vi "MAIN_5.3.vi"() -> ()   [LabVIEW 2012]
doc: "Use this template to build a producer/consumer design pattern with events to produce queue items. Use this design pattern instead of the User Interface Event Handler pattern for user interfaces when you want to execute code asynchronously in response to an event without slowing the user interface responsiveness."
uses:
  State_machine_enum.ctl
  display2.ctl
  User_buttons_enum.ctl
  <vilib>/DAQmx/read.llb/DAQmx Read (Analog 2D DBL NChan NSamp).vi
  Global 1_diag.vi
  <vilib>/Waveform/WDTFileIO.llb/Export Waveforms To Spreadsheet File (1D).vi
  <vilib>/Utility/file.llb/Write To Spreadsheet File (DBL).vi
  <vilib>/DAQmx/create/channels.llb/DAQmx Create Channel (AI-Voltage-Basic).vi
  <vilib>/DAQmx/configure/timing.llb/DAQmx Timing (Sample Clock).vi
  <vilib>/DAQmx/miscellaneous.llb/DAQmx Fill In Error Info.vi
  <vilib>/Analysis/baseanly.llb/Mean (DBL).vi
  <vilib>/express/express arith-compare/Formula/XNode/ExpressFormulaBlockNode.xnode
  <vilib>/Analysis/NI_AALBase.lvlib
  <resource>/objmgr/daqmx.rc
panel:
  out "LD(cont/disc)":T1
  out "LD error array disc":dbl[](array[numeric])
  out "LD array disc":dbl[](array[numeric])
  in  "Timetrace save":bool
  out "result":bool=TRUE
  out "dt":dbl=0.001
  in  "Lock In":bool
  out "dLD_RMS":dbl=nan
  out "Waveform Graph":waveform(dbl)[](graph)=[{"t0"=timestamp(0 s since 1904-01-01), "dt"=0.001, "Y"=[]}, {"t0"=timestamp(0 s since 1904-01-01), "dt"=0.001, "Y"=[]}]
  out "error out":errorcluster
  out "Unbalanced?":bool
  in  "Second Harmonic":bool
  out "path":path
  out "Signal Balance":bool
  out "DC Voltage (V) 2":dbl(knob)=nan scale=0.0..10.0
  out "2f Frequency (Hz)":dbl(knob)=-inf scale=0.0..150.0
  in  "Voltage Divider (10)":bool
  out "Actual Task":string="Plotting"
  out "Motor Voltage (V)":dbl=1.0
  in  "Initial Voltage (V)":dbl=0.35 min=0.0 max=9.0
  in  "Final Voltage (V)":dbl=1.4 min=0.0 max=2.0
  in  "Voltage Step (V)":dbl=0.1 min=0.0 max=1000.0
  in  "Motor Stabilization Time (s)":dbl(knob)=10.0 step=0.001 scale=0.0..30.0
  out "Initial Voltage (V) 2":dbl=1.4 min=0.0 max=9.0
  in  "Final Voltage (V) 2":dbl=4.0 min=0.0 max=2.0
  in  "Voltage Step (V) 2":dbl=0.2 min=0.0 max=1000.0
  in  "Comment (sample no)":string
  in  "Stop Measurement":bool
  in  "Start Measurement Button":bool
  out "Measurement File":path
  in  "New File":bool
  out "Reset?":bool=TRUE
  out "Actual State":T2=enum."Measure"
  in  "Tab Control":T3(tab)=enum."Options"
  in  "Convert mld":bool
  in  "Convert parasiteno":bool
  in  "Convert parasitemia":bool
  in  "Convert cc":bool
  out "MLD (mV/V)":dbl=0.24515589898324114 format="%#_3g"
  out "SA 1f (mv/V)":dbl
  out "Lock_in (mV/V)":dbl
  out "dLock_in (mV/V)":dbl
  out "dMLD (mV/V)":dbl=0.05171335185673877 format="%#_3g"
  out "Phase (deg)":dbl=-68.05035522636679 format="%0.2f"
  out "Phase  dev (deg)":dbl=5.540360076813409 format="%0.2f"
  out "SA 2f (mv/V)":dbl
  out "MLD Amplitude (mV/V)":cluster{dbl[], dbl[]}[](graph)
  in  "dT/T (%)":dbl
  in  "Dilution":dbl=20.0
  in  "Undiluted cc.\n (ng/ml)":dbl
  in  "Undiluted \nParasitemia (%)":dbl format="%#_6f"
  in  "Parasites/ul\nof Blood":dbl
  in  "Convert dT":bool
  in  "MLD (mV/V)":dbl
  out "MLD Phase":cluster{dbl[], dbl[]}(graph)
  out "Down":bool
  out "Up":bool
  out "2f Frequency (Hz)":T4=-inf format="%0.3f"
  out "1f SA (mV/V)":T4 format="%0.3f"
  out "MLD Sim. LIA (mV/V)":T4=nan format="%0.3f"
  out "MLD SA (mV/V)":T4 format="%0.3f"
  in  "Start Scope":bool
  in  "Constant Motor Voltage":dbl=1.0
  in  "Refresh in (s)":i8=1
  in  "stop":bool
  in  "AC?":bool
  out "levelB":dbl format="%#_2g"
  out "levelA":dbl format="%#_3g"
  in  "V/div B":dbl(knob)=0.2 scale=10.0..0.01 scale format="%#_3g"
  in  "level B":dbl(slide) scale=-1.0..1.0 scale format="%#_3g"
  in  "level A":dbl(slide) scale=-1.0..1.0 scale format="%#_3g"
  in  "V/div A":dbl(knob)=0.2 scale=10.0..0.01 scale format="%#.3f"
  out "Oscilloscope":waveform(dbl)[](graph)=[{"t0"=timestamp(0 s since 1904-01-01), "dt"=0.001, "Y"=[]}, {"t0"=timestamp(0 s since 1904-01-01), "dt"=0.001, "Y"=[]}]
  in  "Sensitivity":T5(ring)
  in  "samples per channel":i32=1000
  in  "rate":dbl=1000.0 format="%0.2f"
  out "Spectrum (mVRMS/Vdc)":cluster{"f0":dbl, "df":dbl, "magnitude":dbl[]}(graph)={"f0"=0.0, "df"=inf, "magnitude"=[]}
  out "MLD LIA (mV/V)":dbl=0.0123978
  out "Lockin_freq":dbl=9.4676
  out "DC Voltage (V)":T4=nan format="%0.3f"
  out "Time Domain Signal":cluster{"xi used":dbl[], "yi":dbl[]}[](graph)
  out "Signal Spectrum (mVrms/Vdc)":cluster{"f0":dbl, "df":dbl, "magnitude":dbl[]}[](graph)
  out "1f 2f Spectral Peaks":T6
  out "Lock-in R (Vrms)":cluster{dbl[], "Result":dbl[]}(graph)
  out "Lock-in Theta":cluster{dbl[], "Result":dbl[]}(graph)
  in  "Pike Removal (StDev)":dbl=3.0
  in  "Lock-in Time (s)":dbl=10.0
  in  "dt (s)":dbl=0.0002
  in  "Resolution (s)":dbl=0.0001
  in  "Averaging time (s)":dbl=1.0 format="%0.2p"
  in  "Cutoff Frequency (Hz)":dbl=500.0
  in  "Rate":dbl=5000.0 caption="Sample Rate (Hz)" format="%0.2f"
  in  "Samples per Channel":i32=100000
  out "Minimum Value":dbl=-1.0 caption="LD min Value (V)" format="%0.2f"
  out "Maximum Value":dbl=1.0 caption="LD max Value (V)" format="%0.2f"
  in  "DC # samples":i32=100
  in  "DC Sampling Rate (Hz)":dbl=100.0
  in  "Dc min":dbl format="%0.2f"
  in  "Dc max":dbl=10.0 format="%0.2f"
  in  "Reference Signal":tag="Dev3/ai1"
  in  "LD Signal":tag="Dev3/ai0" caption="LD Channel"
  in  "DC Voltage DAQ":tag="Dev3/ai2"
  in  "Motor Channel":tag="Dev3/ao1"
  in  "Lock-in-Amplifier VISA":refnum<visa-resource-name>="GPIB0::3::INSTR"
  out "Dc standard deviation":dbl=-0.0 format="%0.2f"
  out "Dc mean":dbl=nan format="%0.2f"
  out "dPhase array":dbl[](array[numeric])
  out "Phase array":dbl[](array[numeric])
  out "LD array":dbl[](array[numeric])
  out "Frequency array":dbl[](array[numeric])
  out "LD error array":dbl[](array[numeric])
  out "First?":bool
  out "Stopped":bool
  out "Last Step?":bool
  in  "EXIT":bool
  # "Measurement Settings"
  # "Motor Setup"
  # "OFF"
  # "ON"
  # "Actual Datapoint Values"
  # "Convert quantities"
  # "Physical channels"
  # "Signal Processing Settings"
  # "DC Acquisition Settings"
  # "LD Acquisition Settings"
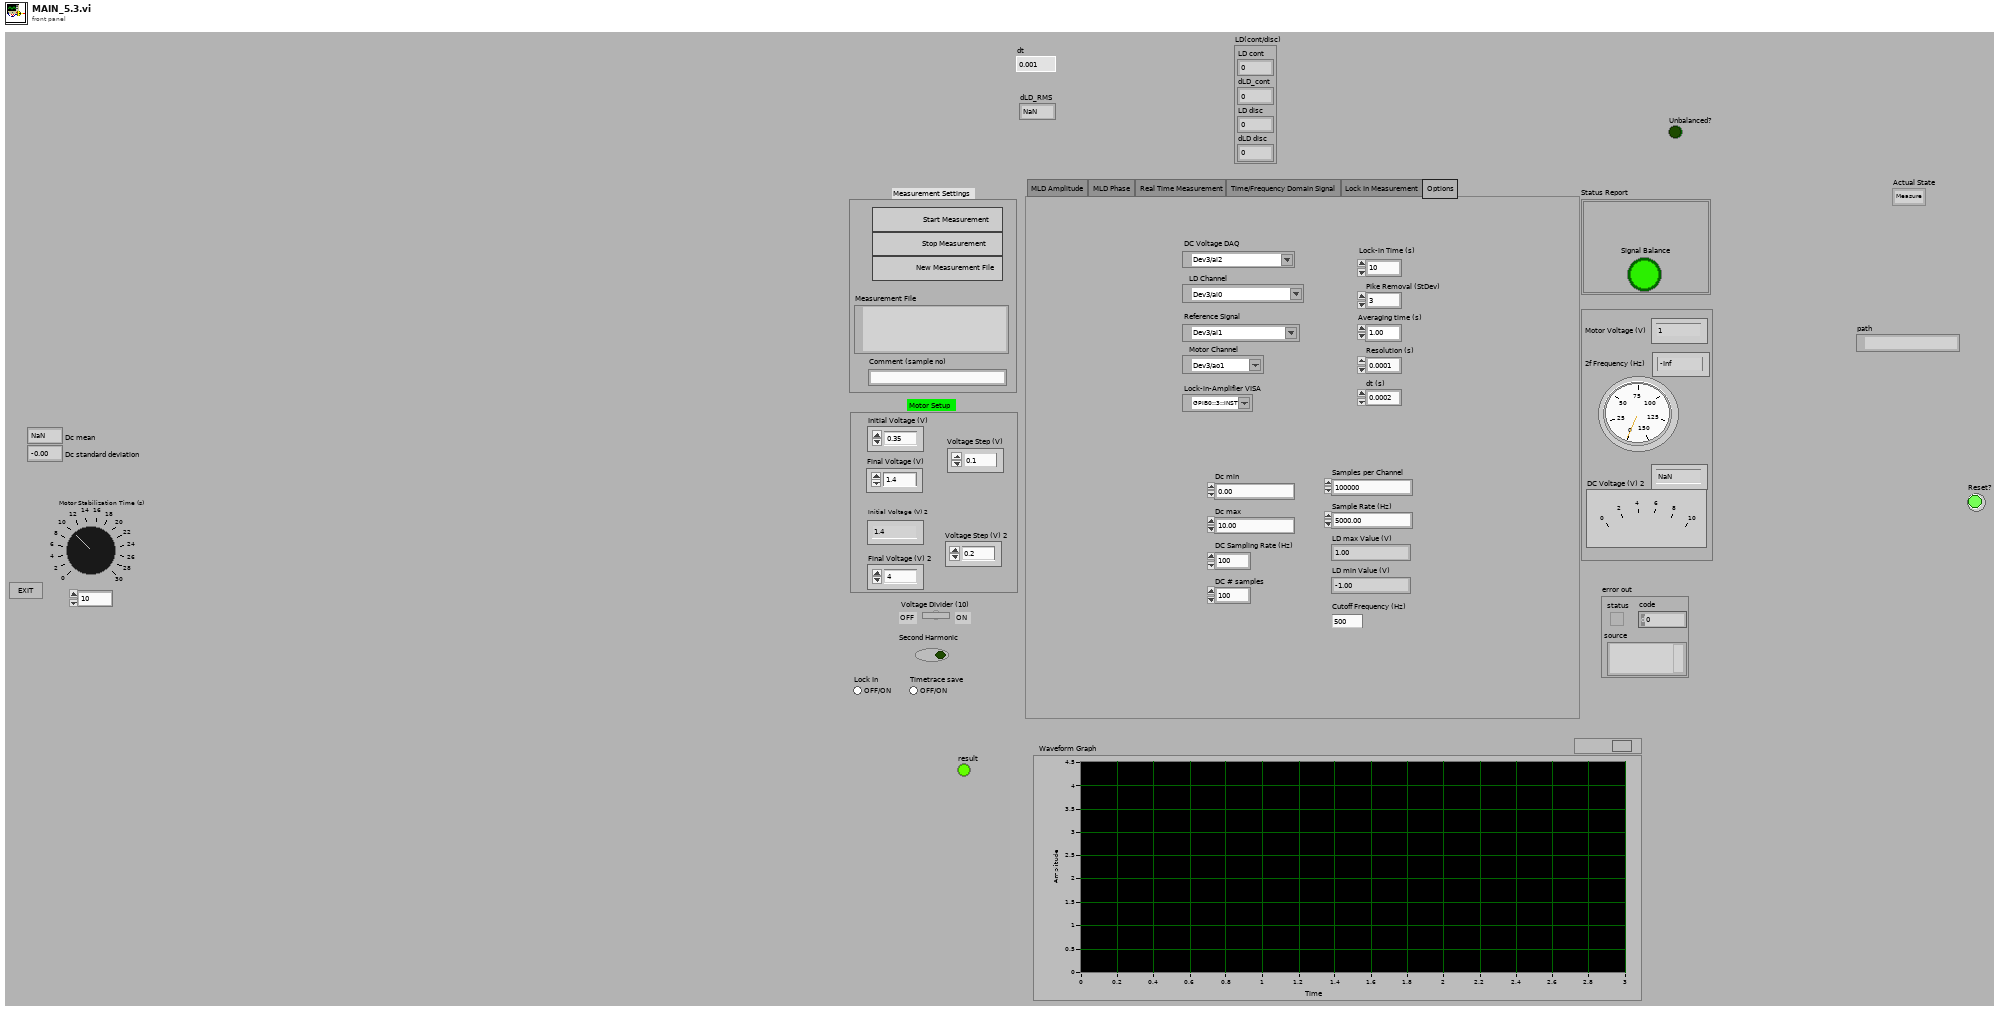
[diagram p1: front panel]
types:
  T1 = cluster{"LD cont":dbl, "dLD_cont":dbl, "LD disc":dbl, "dLD disc":dbl}
  T2 = typedef "State_machine_enum.ctl" = enum16{"SetMotor", "Stabilize", "Measure", "Process", "Save", "Finished"}
  T3 = enum32{"MLD Amplitude", "MLD Phase", "Real Time Measurement", "Time/Frequency Domain Signal", "Lock In Measurement", "Options"}
  T4 = typedef "display2.ctl" = dbl
  T5 = enum16{"-1V..1V", "-1.25V..1.25V", "-2V..2V", "-2.5V..2.5V", "-4V..4V", "-5V..5V", "-10V..10V"}
  T6 = cluster{"1f (Hz)":dbl, "U1f (mV/V)":dbl, "2f (Hz)":dbl, "U2f (mV/V)":dbl}
  T7 = typedef "User_buttons_enum.ctl" = enum16{"start", "stop", "exit", "New", "Scope", "Continue"}
  T8 = enum16{"open", "replace", "create", "open or create", "replace or create", "replace or create with confirmation"}
  T9 = enum16{"Left Button", "Center Button", "Right Button", "Window Close"}
  T10 = cluster{dbl, "1f Ampl (Vrms/Vdc)":dbl, dbl, "2f Ampl (Vrms/Vdc)":dbl}
  T11 = cluster{"Frequency array":dbl[], "LD array disc":dbl[]}
  T12 = cluster{"Frequency array":dbl[], "LD array":dbl[]}
  T13 = cluster{"Frequency array":dbl[], "Phase array":dbl[]}
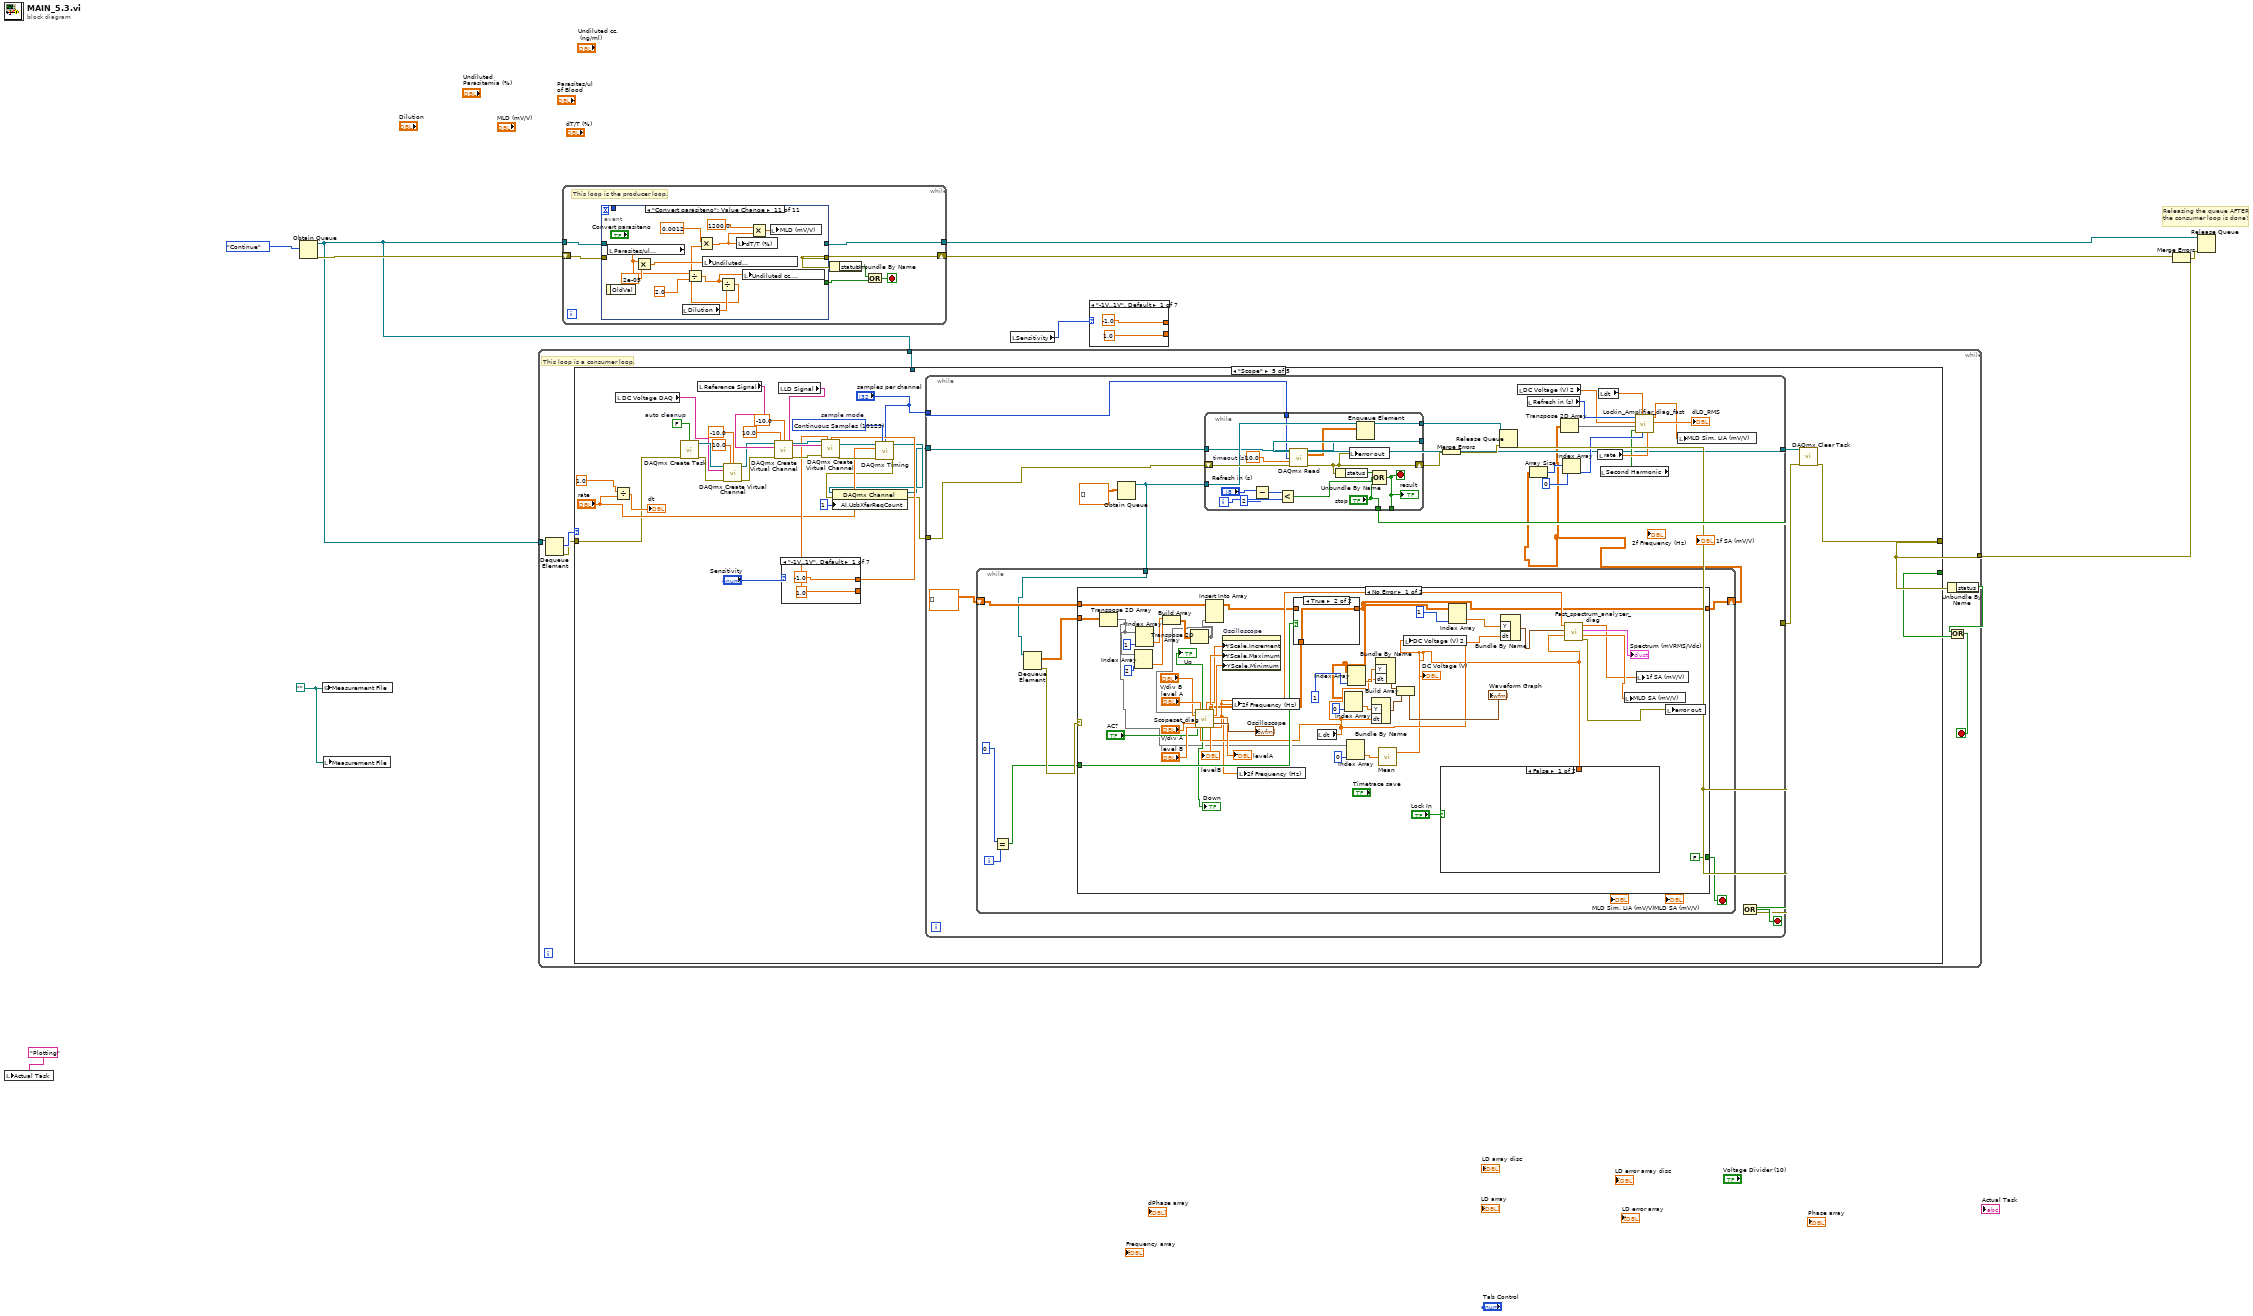
[diagram p0: block diagram]
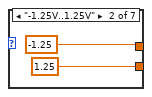
[diagram p2: hidden frame]
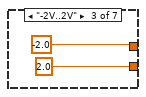
[diagram p3: hidden frame]
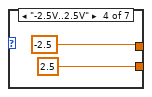
[diagram p4: hidden frame]
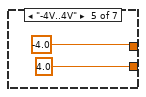
[diagram p5: hidden frame]
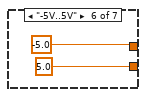
[diagram p6: hidden frame]
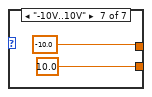
[diagram p7: hidden frame]
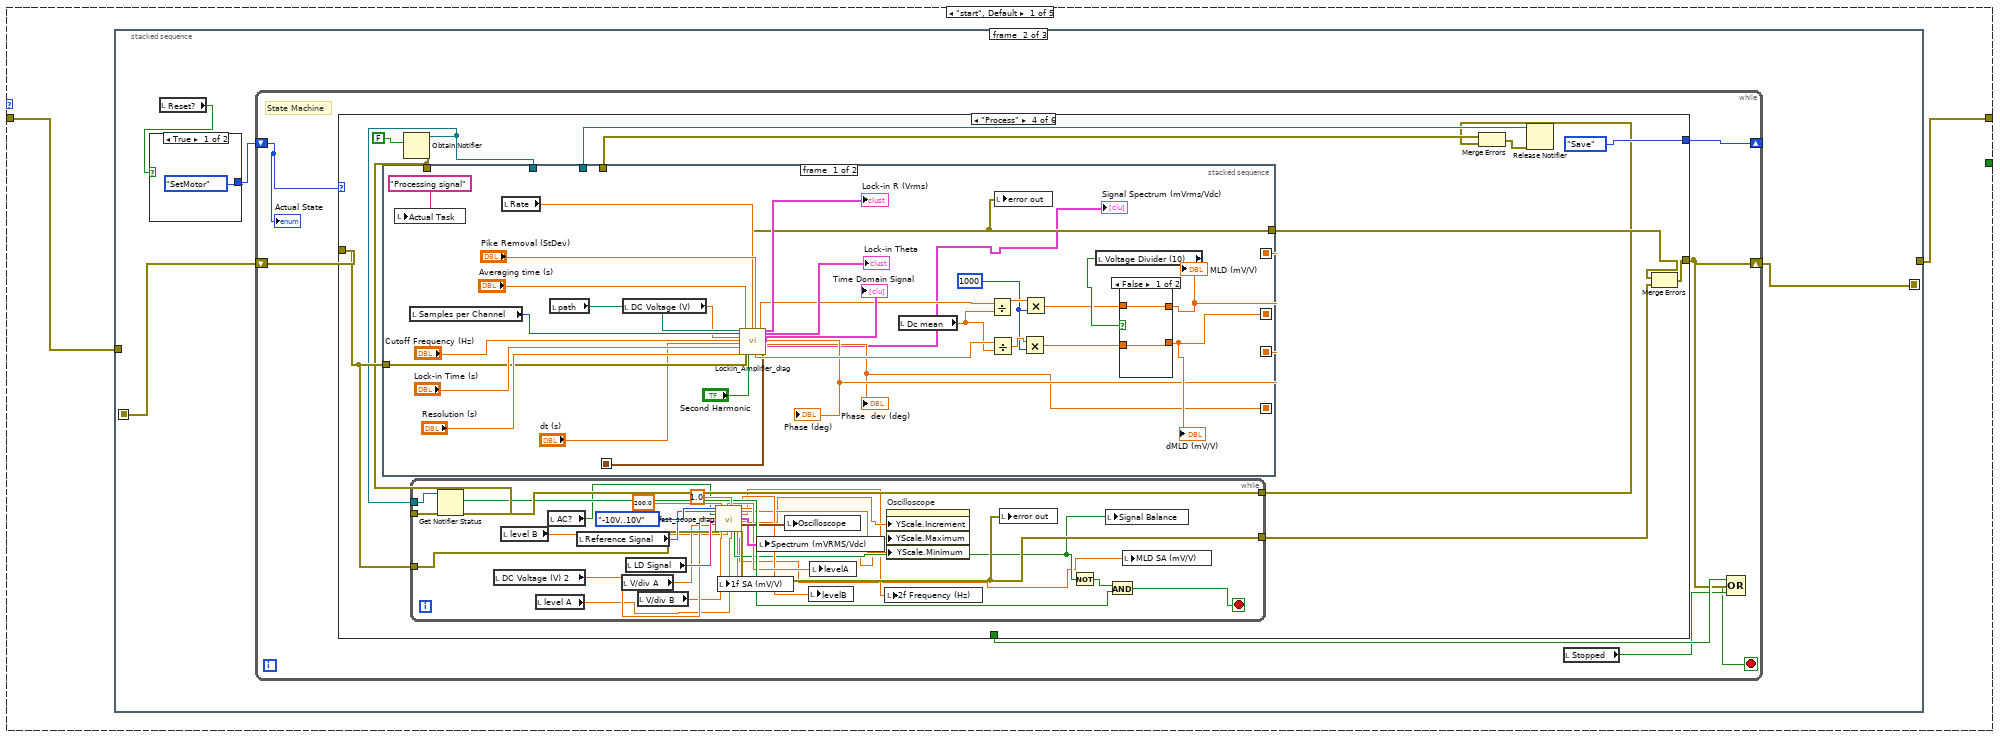
[diagram p8: hidden frame]
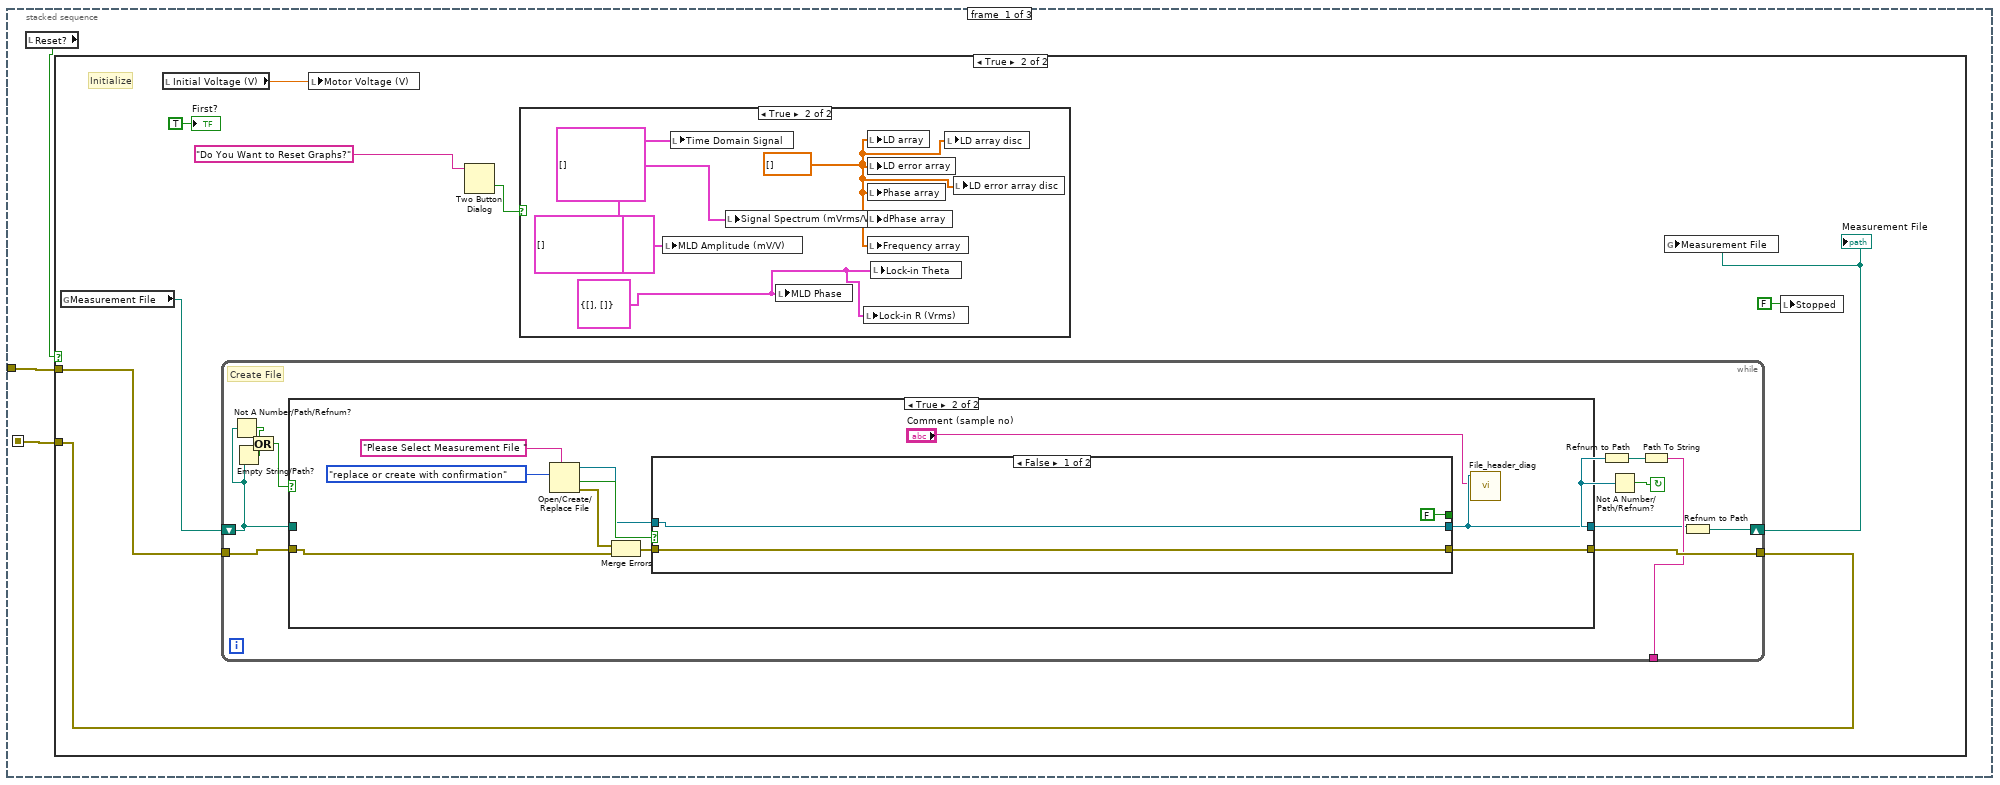
[diagram p9: hidden frame]
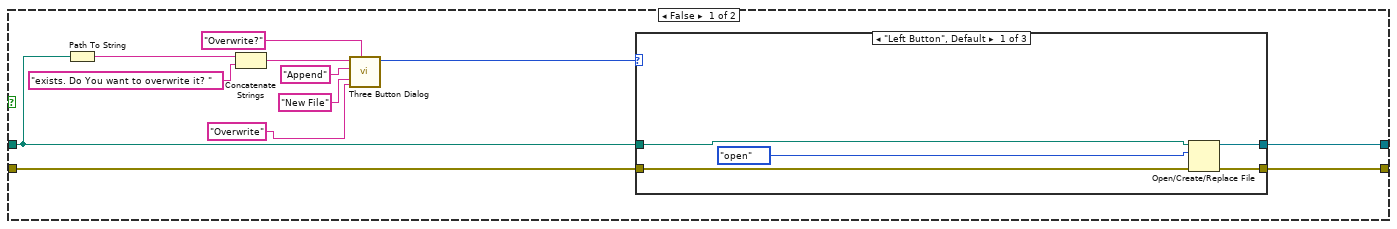
[diagram p11: hidden frame]
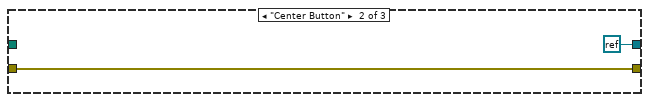
[diagram p12: hidden frame]
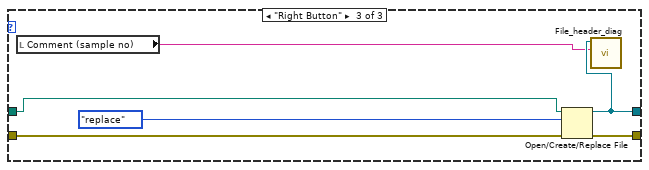
[diagram p13: hidden frame]
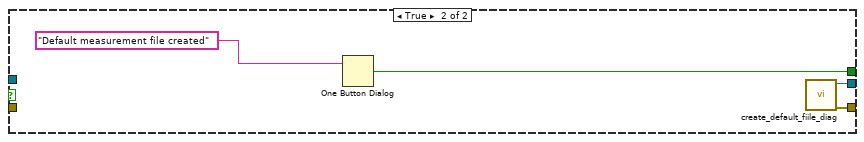
[diagram p14: hidden frame]
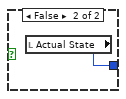
[diagram p16: hidden frame]
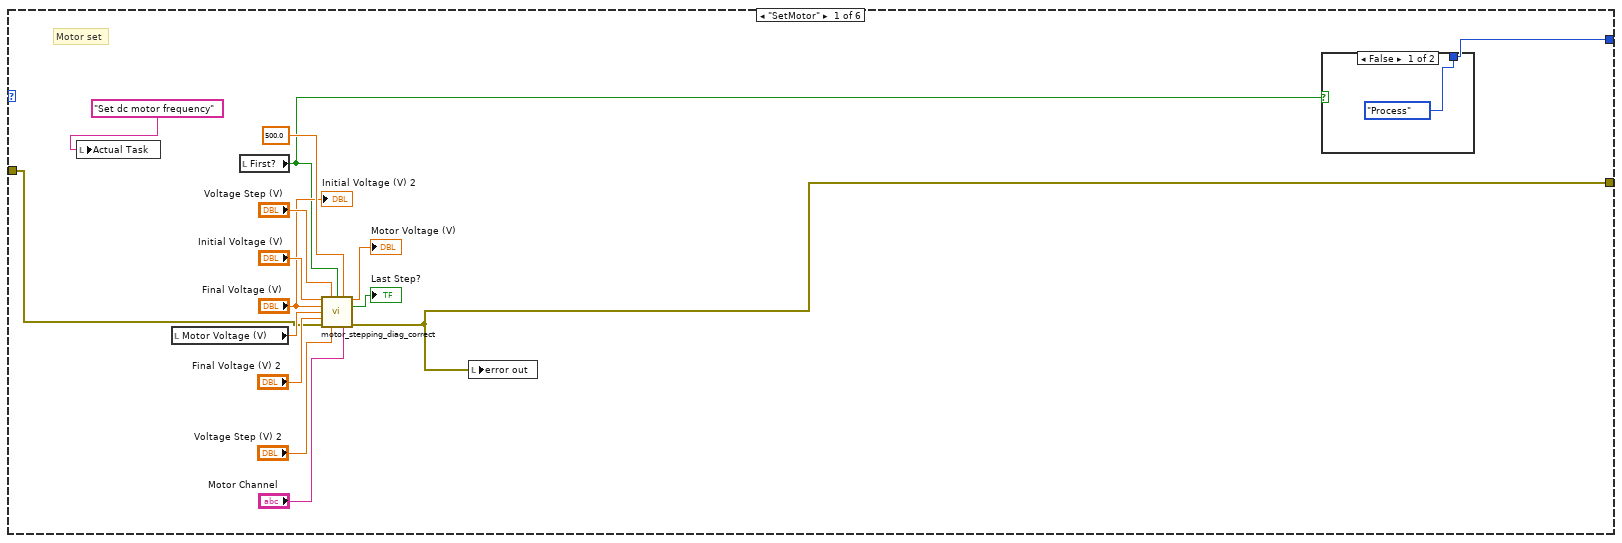
[diagram p17: hidden frame]
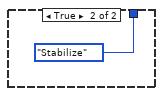
[diagram p18: hidden frame]
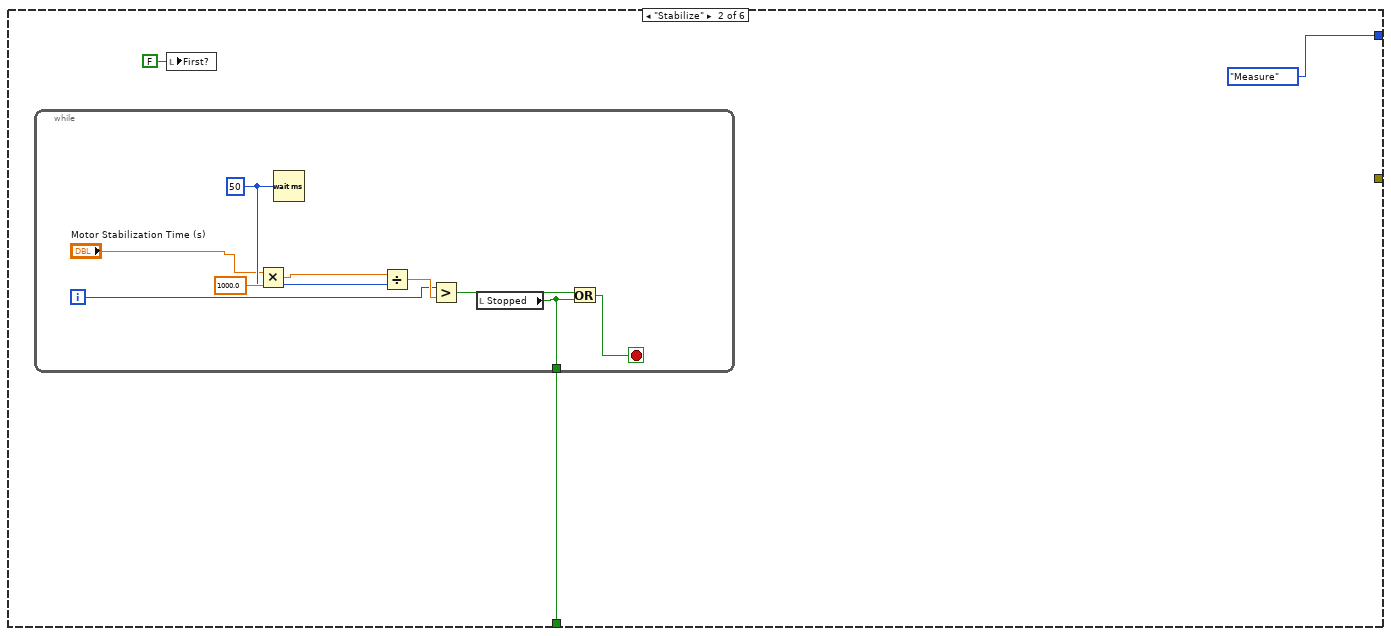
[diagram p19: hidden frame]
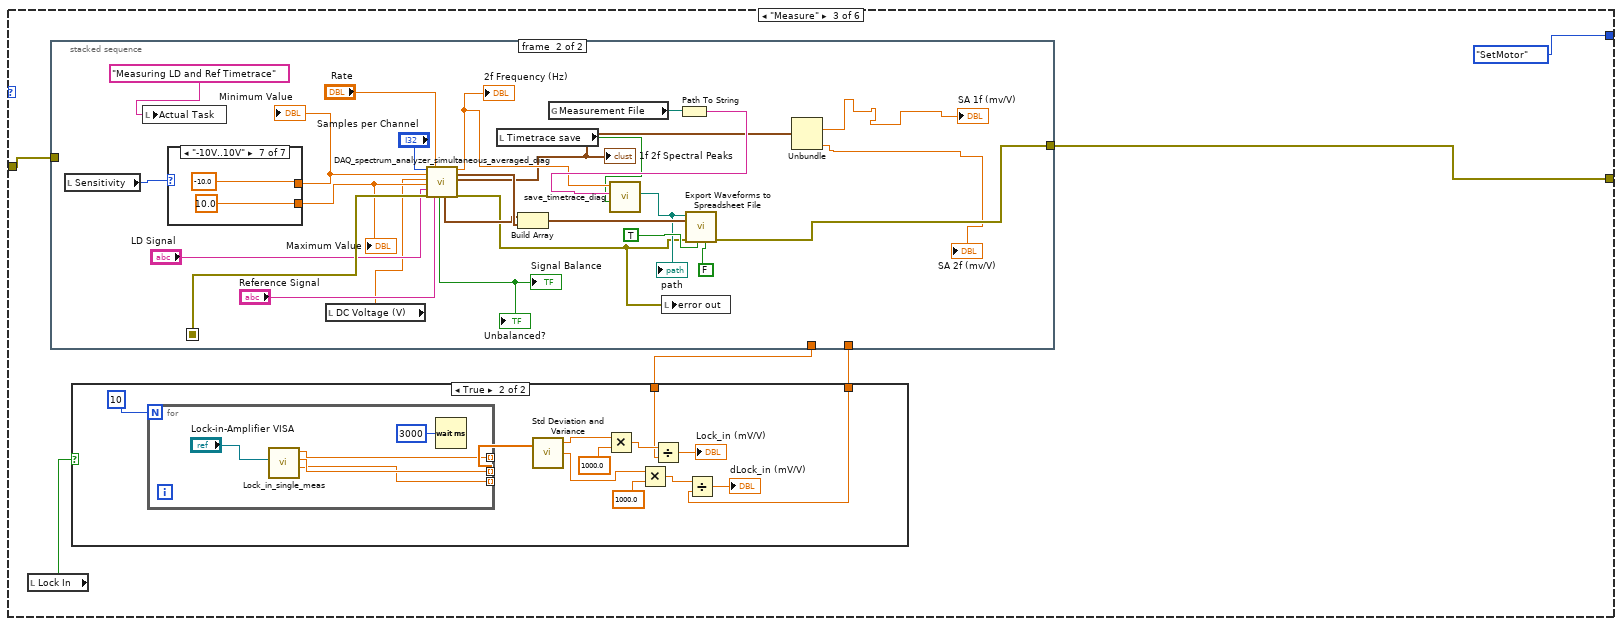
[diagram p20: hidden frame]
diagram:
  w4 = path ""
  # "Releasing the queue AFTER\nthe consumer loop is done!"
  n1 = local write "Actual Task"("Plotting" ("Actual Task")) -> ()
  n2 = Obtain Queue(element data type=User_buttons_enum."Continue") -> (queue out=w3:refnum<queue>, error out=w10:errorcluster)  [unwired: 4 in, 1 out]
  n3 = global write "Global 1_diag.vi" "Measurement File"(w4) -> ()
  n4 = local write "Measurement File"(w4) -> ()
  n5 = while {
    tunnel: w3 -> [w18]
    tunnel: [w15] -> w6
    tunnel: w3 -> [w11]
    stop <- w12 stop-if-true
    # "This loop is a consumer loop."
    n6 = Dequeue Element(queue=w18) -> (element=w17:T7, error out=w16:errorcluster)  [unwired: 2 in, 2 out]
    n7 = case shown="\"Scope\"" w17 {
      tunnel: [_ _ TRUE _ _] -> w13
      tunnel: w16 -> [w20 w373 w435 w439 w447]
      tunnel: [w19 w372 w435 w438 w453] -> w15
      tunnel: w11 -> [_ w371 _ _ _]
      frame "start", Default {
        n8 = stacked-sequence {
          seq-local: [w22 _ _] -> [_ w95 _]
          seq-local: [_ w94 _] -> [_ _ w358]
          tunnel: w20 -> [w23 _ w356]
          tunnel: [_ _ w355] -> w19
          frame #0 {
            n9 = local read "Reset?"() -> (w21:bool)
            n10 = case shown="True" w21 {
              tunnel: w23 -> [w24 w28]
              tunnel: [w24 w26] -> w22
              frame False {
              }
              frame True {
                # "Initialize"
                n11 = global read "Global 1_diag.vi" "Measurement File"() -> (w27:path)
                n12 = local read "Initial Voltage (V)"() -> (w31:dbl)
                n13 = while {
                  tunnel: [w44] -> w26
                  tunnel: w28 -> [w43]
                  shift-right: [w38] -> w25
                  shift-left: w27 -> [w37]
                  tunnel: [w40] -> _
                  stop <- w42 continue-if-true
                  # "Create File"
                  n14 = Not A Number/Path/Refnum?(number/path/refnum=w37) -> (NaN/Path/Refnum?=w36:bool)
                  n15 = Empty String/Path?(string/path=w37) -> (empty?=w35:bool)
                  n16 = Or(x=w36, y=w35) -> (x .or. y?=w34:bool)
                  n17 = case shown="True" w34 {
                    tunnel: [w51 w72] -> w39
                    tunnel: [w50 w71] -> w44
                    tunnel: w43 -> [w49 w73]
                    tunnel: w37 -> [w45 _]
                    frame False {
                      n18 = Path To String(path=w45) -> (string=w48:string)
                      n19 = Concatenate Strings(w48, "exists. Do You want to overwrite it? " ("message")) -> (w46:string)
                      n20 = call <vilib>:"Three Button Dialog.vi"("Window Title (\"\")"="Overwrite?" ("Window Title (\"\")"), "Right Button Text (\"Cancel\")"="Overwrite" ("Right Button Text (\"Cancel\")"), "Center Button Text (\"No\")"="New File" ("Center Button Text (\"No\")"), "Left Button Text (\"Yes\")"="Append" ("Left Button Text (\"Yes\")"), "message"=w46) -> ("Which Button?"=w52:T9)  [unwired: 6 in]
                      n21 = case shown="\"Left Button\", Default" w52 {
                        tunnel: w45 -> [w57 _ w65]
                        tunnel: [w58 refnum<k0> refnum w66] -> w51
                        tunnel: [w60 w62 w68] -> w50
                        tunnel: w49 -> [w59 w62 w67]
                        frame "Left Button", Default {
                          n22 = Open/Create/Replace File(file path (use dialog)=w57, error in=w59, operation (0:open)=T8."open") -> (refnum out=w58:refnum<file>, error out=w60:errorcluster)  [unwired: 3 in, 1 out]
                        }
                        frame "Center Button" {
                        }
                        frame "Right Button" {
                          n23 = local read "Comment (sample no)"() -> (w64:string)
                          n24 = Open/Create/Replace File(file path (use dialog)=w65, error in=w67, operation (0:open)=T8."replace") -> (refnum out=w66:refnum<file>, error out=w68:errorcluster)  [unwired: 3 in, 1 out]
                          n25 = call "File_header_diag.vi"("Comment"=w64, "Byte Stream File in"=w66) -> ()  [unwired: 10 in]
                        }
                      }
                    }
                    frame True {
                      n26 = Open/Create/Replace File(prompt="Please Select Measurement File ", operation (0:open)=T8."replace or create with confirmation") -> (refnum out=w76:refnum<file>, cancelled=w77:bool, error out=w75:errorcluster)  [unwired: 4 in]
                      n27 = Merge Errors(w75, w73) -> (w74:errorcluster)
                      n28 = case shown="False" w77 {
                        tunnel: w76 -> [w82 _]
                        tunnel: [w82 w83] -> w72
                        tunnel: [w81 w85] -> w71
                        tunnel: w74 -> [w81 _]
                        tunnel: [FALSE ("true") w84] -> _
                        frame False {
                        }
                        frame True {
                          n29 = One Button Dialog(message="Default measurement file created") -> (true=w84:bool)  [unwired: 1 in]
                          n30 = call "create_default_fiile_diag.vi"() -> ("error out"=w85:errorcluster, "Byte Stream File out"=w83:refnum<file>)  [unwired: 10 in]
                        }
                      }
                      n31 = call "File_header_diag.vi"("Comment"="Comment (sample no)", "Byte Stream File in"=w72) -> ()  [unwired: 10 in]
                    }
                  }
                  n32 = Refnum to Path(1:w39) -> (0:w41:path)
                  n33 = Not A Number/Path/Refnum?(number/path/refnum=w39) -> (NaN/Path/Refnum?=w42:bool)
                  n34 = Path To String(path=w41) -> (string=w40:string)
                  n35 = Refnum to Path(1:w39) -> (0:w38:path)
                }
                "Measurement File" <- w25
                n36 = local write "Motor Voltage (V)"(w31) -> ()
                n37 = Two Button Dialog(message="Do You Want to Reset Graphs?") -> (T button?=w29:bool)  [unwired: 2 in]
                n38 = case shown="True" w29 {
                  frame False {
                  }
                  frame True {
                    w88 = cluster{"magnitude":dbl[], "magnitude 2":dbl[]} {"magnitude"=[], "magnitude 2"=[]} ("MLD Amplitude")
                    w87 = dbl[] []
                    n39 = local write "MLD Amplitude (mV/V)"(cluster{dbl[], dbl[]}[] [] ("MLD Amplitude (mV/V)")) -> ()
                    n40 = local write "Time Domain Signal"(cluster{dbl[], dbl[]}[] [] ("Integral")) -> ()
                    n41 = local write "Signal Spectrum (mVrms/Vdc)"(cluster{"f0":dbl, "df":dbl, dbl[]}[] [] ("Signal Spectrum")) -> ()
                    n42 = local write "MLD Phase"(w88) -> ()
                    n43 = local write "Lock-in R (Vrms)"(w88) -> ()
                    n44 = local write "LD array"(w87) -> ()
                    n45 = local write "LD error array"(w87) -> ()
                    n46 = local write "Phase array"(w87) -> ()
                    n47 = local write "dPhase array"(w87) -> ()
                    n48 = local write "Frequency array"(w87) -> ()
                    n49 = local write "Lock-in Theta"(w88) -> ()
                    n50 = local write "LD array disc"(w87) -> ()
                    n51 = local write "LD error array disc"(w87) -> ()
                  }
                }
                n52 = global write "Global 1_diag.vi" "Measurement File"(w25) -> ()
                n53 = local write "Stopped"(FALSE ("Stopped")) -> ()
                "First?" <- TRUE ("First?")
              }
            }
          }
          frame #1 {
            n54 = local read "Reset?"() -> (w92:bool)
            n55 = case shown="True" w92 {
              tunnel: [State_machine_enum."SetMotor" w97] -> w93
              frame True {
              }
              frame False {
                n56 = local read "Actual State"() -> (w97:T2)
              }
            }
            n57 = while {
              shift-right: [w98] -> _
              shift-left: w93 -> [w104]
              shift-right: [w102] -> w94
              shift-left: w95 -> [w99]
              stop <- w100 stop-if-true
              # "State Machine"
              n58 = case shown="\"Process\"" w104 {
                tunnel: [w112 _ w139 w217 w335 _] -> w102
                tunnel: [_ w124 _ _ _ w354] -> w103
                tunnel: w99 -> [w113 _ w138 w215 w335 _]
                tunnel: [w118 State_machine_enum."Measure" State_machine_enum."SetMotor" State_machine_enum."Save" w334 State_machine_enum."SetMotor"] -> w98
                frame "SetMotor" {
                  # "Motor set"
                  n59 = local write "Actual Task"("Set dc motor frequency" ("Actual Task")) -> ()
                  n60 = local read "Motor Voltage (V)"() -> (w115:dbl)
                  n61 = local read "First?"() -> (w105:bool)
                  n62 = call "motor_stepping_diag_correct.vi"("Initial Voltage (V)"="Initial Voltage (V)", "Voltage Step (V)"="Voltage Step (V)", "First?"=w105, "Steps"=500.0, "Final Voltage (V)"="Final Voltage (V)", "Actual Voltage (V)  in"=w115, "Final Voltage (V) 2"="Final Voltage (V) 2", "error in (no error)"=w113, "Voltage Step2"="Voltage Step (V) 2", "Physical Channel"="Motor Channel") -> ("Actual Voltage (V)"=→"Motor Voltage (V)":dbl, "Boolean"=→"Last Step?":bool, "error out"=w112:errorcluster)  [unwired: 3 in]
                  n63 = local write "error out"(w112) -> ()
                  n64 = case shown="False" w105 {
                    tunnel: [State_machine_enum."Process" State_machine_enum."Stabilize"] -> w118
                    frame False {
                    }
                    frame True {
                    }
                  }
                  "Initial Voltage (V) 2" <- "Final Voltage (V)"
                }
                frame "Stabilize" {
                  n65 = while {
                    tunnel: [w125] -> w124
                    i -> [w126]
                    stop <- w128 stop-if-true
                    w131 = u32 50 ("milliseconds to wait")
                    n66 = Multiply(x="Motor Stabilization Time (s)", y=1000.0) -> (x*y=w133:dbl)
                    n67 = Wait (ms)(milliseconds to wait=w131) -> ()  [unwired: 1 out]
                    n68 = Divide(x=w133, y=w131) -> (x/y=w130:dbl)
                    n69 = Greater?(x=w126, y=w130) -> (0:w129:bool)
                    n70 = local read "Stopped"() -> (w125:bool)
                    n71 = Or(x=w129, y=w125) -> (x .or. y?=w128:bool)
                  }
                  n72 = local write "First?"(FALSE ("First?")) -> ()
                }
                frame "Measure" {
                  n73 = local read "Lock In"() -> (w134:bool)
                  n74 = stacked-sequence {
                    seq-local: [w162 _] -> [_ w194]
                    tunnel: [_ w193] -> w139
                    tunnel: w138 -> [w158 _]
                    tunnel: [w157 _] -> w137
                    tunnel: [w157 _] -> w136
                    frame #0 {
                      n75 = local write "Actual Task"("Measuring DC Voltage" ("Actual Task")) -> ()
                      n76 = call "manualDAQ_diag.vi"("minimum value"="Dc min", "Rate"="DC Sampling Rate (Hz)", "error in (no error)"=w158, "Samples per Channel"="DC # samples", "maximum value"="Dc max", "physical channels"="DC Voltage DAQ") -> ("error out"=w162:errorcluster, "output waveform"=w164:waveform(dbl))  [unwired: 4 in]
                      "error out" <- w162
                      n77 = Unbundle By Name(w164) -> ("Y"=w165:dbl[])
                      n78 = call <vilib>:"Std Deviation and Variance.vi"("X"=w165) -> ("mean"=w157:dbl, "standard deviation"=→"Dc standard deviation":dbl)  [unwired: 1 in, 1 out]
                      "DC Voltage (V) 2" <- w157
                      "Dc mean" <- w157
                      n79 = local write "DC Voltage (V)"(w157) -> ()
                    }
                    frame #1 {
                      n80 = local read "Sensitivity"() -> (w174:T5)
                      n81 = local write "Actual Task"("Measuring LD and Ref Timetrace" ("Actual Task")) -> ()
                      n82 = case shown="\"-10V..10V\"" w174 {
                        tunnel: [-1.0 ("maximum value") -1.25 ("maximum value") -2.0 ("maximum value") -2.5 ("maximum value") -4.0 ("maximum value") -5.0 ("maximum value") -10.0 ("maximum value")] -> w173
                        tunnel: [1.0 ("maximum value") 1.25 ("maximum value") 2.0 ("maximum value") 2.5 ("maximum value") 4.0 ("maximum value") 5.0 ("maximum value") 10.0 ("maximum value")] -> w172
                        frame "-1V..1V", Default {
                        }
                        frame "-1.25V..1.25V" {
                        }
                        frame "-2V..2V" {
                        }
                        frame "-2.5V..2.5V" {
                        }
                        frame "-4V..4V" {
                        }
                        frame "-5V..5V" {
                        }
                        frame "-10V..10V" {
                        }
                      }
                      "Maximum Value" <- w172
                      "Minimum Value" <- w173
                      n83 = local read "DC Voltage (V)"() -> (w171:T4)
                      n84 = call "DAQ_spectrum_analyzer_simultaneous_averaged_diag.vi"("Samples per Channel"="Samples per Channel", "minimum value"=w173, "DC voltage (V)"=w171, "maximum value"=w172, "LD channel"="LD Signal", "Error In"=w194, "Rate"="Rate", "Ref channel"="Reference Signal") -> ("Unbalanced?"=→"Signal Balance" →"Unbalanced?":bool, "raw signal waveform"=w180:waveform(dbl), "Calculated frequency"=w182:dbl, "Reference Timetrace"=w181:waveform(dbl), "1f 2f"=w179:T10, "error out"=w176:errorcluster)  [unwired: 1 in, 5 out]
                      "2f Frequency (Hz)" <- w182
                      "1f 2f Spectral Peaks" <- w179
                      n85 = local read "Timetrace save"() -> (w175:bool)
                      n86 = Build Array(w180, w181) -> (w183:waveform(dbl)[])
                      n87 = global read "Global 1_diag.vi" "Measurement File"() -> (w185:path)
                      n88 = local write "error out"(w176) -> ()
                      n89 = Path To String(path=w185) -> (string=w184:string)
                      n90 = call "save_timetrace_diag.vi"("Boolean"=w175, "FilaPath"=w184, "Numeric"=w182) -> ("path"=w178:path)  [unwired: 7 in, 1 out]
                      "path" <- w178
                      n91 = call-poly <vilib>:"Export Waveforms to Spreadsheet File.vi"("header? (write header:T)"=FALSE, "append to file? (new file:F)"=TRUE ("header? (write header:T)"), "error in (no error)"=w176, "waveforms"=w183, "file path (dialog if empty)"=w178) -> ("error out"=w193:errorcluster)  [unwired: 5 in, 1 out]
                      n92 = Unbundle(w179) -> ("1f Ampl (Vrms/Vdc)"=→"SA 1f (mv/V)":dbl, "2f Ampl (Vrms/Vdc)"=→"SA 2f (mv/V)":dbl)  [unwired: 2 out]
                    }
                  }
                  n93 = case shown="True" w134 {
                    tunnel: w137 -> [_ w146]
                    tunnel: w136 -> [_ w142]
                    frame False {
                    }
                    frame True {
                      n94 = for {
                        N: 10 -> [_]
                        tunnel: [w154] -> _ mode=indexing
                        tunnel: [w153] -> w150 mode=indexing
                        tunnel: [w152] -> _ mode=indexing
                        n95 = call "Lock_in_single_meas.vi"("Lock-in-Amplifier VISA"="Lock-in-Amplifier VISA") -> ("Lockin_phas"=w152:dbl, "Lockin_ampl"=w153:dbl, "Freq"=w154:dbl)  [unwired: 7 in, 1 out]
                        n96 = Wait (ms)(milliseconds to wait=u32 3000) -> ()  [unwired: 1 out]
                      }
                      n97 = call <vilib>:"Std Deviation and Variance.vi"("X"=w150) -> ("mean"=w149:dbl, "standard deviation"=w143:dbl)  [unwired: 1 in, 1 out]
                      n98 = Multiply(x=w149, y=1000.0) -> (x*y=w147:dbl)
                      n99 = Multiply(x=w143, y=1000.0) -> (x*y=w145:dbl)
                      n100 = Divide(x=w147, y=w146) -> (x/y=→"Lock_in (mV/V)":dbl)
                      n101 = Divide(x=w145, y=w142) -> (x/y=→"dLock_in (mV/V)":dbl)
                    }
                  }
                }
                frame "Process" {
                  n102 = Obtain Notifier(notification data type=FALSE) -> (notifier out=w211:refnum<notifier>, error out=w210:errorcluster)  [unwired: 3 in, 1 out]
                  n103 = stacked-sequence {
                    seq-local: [w261 _] -> [_ w316]
                    seq-local: [w260 _] -> [_ w315]
                    seq-local: [w259 _] -> [_ w314]
                    seq-local: [w258 _] -> [_ w313]
                    seq-local: [w251 _] -> [_ w307]
                    tunnel: w215 -> [w271 _]
                    tunnel: [w256 _] -> w219
                    tunnel: w211 -> [_ w312]
                    tunnel: [_ w310] -> w214
                    tunnel: w210 -> [_ w309]
                    tunnel: [_ w308] -> w212
                    frame #0 {
                      w255 = 1000
                      n104 = local write "Actual Task"("Processing signal" ("Actual Task")) -> ()
                      n105 = local read "Samples per Channel"() -> (w281:i32)
                      n106 = local read "Rate"() -> (w272:dbl)
                      n107 = local read "path"() -> (w270:path)
                      n108 = local read "DC Voltage (V)"() -> (w252:T4)
                      n109 = call "Lockin_Amplifier_diag.vi"("Reference signal (dialog if empty)"=w270, "Sample Number"=w281, "DC(V)"=w252, "Cutoff Frequency"="Cutoff Frequency (Hz)", "dt"="dt (s)", "Window (s)"="Lock-in Time (s)", "Resolution"="Resolution (s)", "averaging time"="Averaging time (s)", "Error In"=w271, "Second"="Second Harmonic", "Sampling Freq"=w272, "tolerance (Deviation)"="Pike Removal (StDev)") -> ("Error Out"=w256:errorcluster, "dLD_RMS"=w264:dbl, "LD_RMS"=w262:dbl, "Signal Spectrum"=→"Signal Spectrum (mVrms/Vdc)":cluster{"f0":dbl, "df":dbl, "magnitude":dbl[]}[], "LD(cont/disc)"=w251:T1, "Lock-in R (Vrms)"=→"Lock-in R (Vrms)":cluster{dbl[], "Result":dbl[]}, "Lock-in Theta"=→"Lock-in Theta":cluster{dbl[], "Result":dbl[]}, "Time Domain Signal"=→"Time Domain Signal":cluster{"xi used":dbl[], "yi":dbl[]}[], "Phase average"=w259:dbl, "Phase  deviation"=w258:dbl)  [unwired: 4 in, 2 out]
                      "Phase (deg)" <- w259
                      "Phase  dev (deg)" <- w258
                      n110 = local read "Dc mean"() -> (w254:dbl)
                      n111 = Divide(x=w262, y=w254) -> (x/y=w269:dbl)
                      n112 = Divide(x=w264, y=w254) -> (x/y=w268:dbl)
                      n113 = local write "error out"(w256) -> ()
                      n114 = Multiply(x=w268, y=w255) -> (x*y=w265:dbl)
                      n115 = Multiply(x=w269, y=w255) -> (x*y=w266:dbl)
                      n116 = local read "Voltage Divider (10)"() -> (w267:bool)
                      n117 = case shown="False" w267 {
                        tunnel: w266 -> [w284 w289]
                        tunnel: w265 -> [w283 w288]
                        tunnel: [w284 w286] -> w261
                        tunnel: [w283 w285] -> w260
                        frame False {
                        }
                        frame True {
                          w287 = 10
                          n118 = Multiply(x=w289, y=w287) -> (x*y=w286:dbl)
                          n119 = Multiply(x=w288, y=w287) -> (x*y=w285:dbl)
                        }
                      }
                      "MLD (mV/V)" <- w261
                      "dMLD (mV/V)" <- w260
                    }
                    frame #1 {
                      w296 = 1000
                      n120 = Unbundle(w307) -> ("LD disc"=w294:dbl, "dLD disc"=w293:dbl)  [unwired: 2 out]
                      n121 = local read "LD error array disc"() -> (w305:dbl[])
                      n122 = local read "Dc mean"() -> (w295:dbl)
                      n123 = local read "LD array disc"() -> (w306:dbl[])
                      n124 = Divide(x=w294, y=w295) -> (x/y=w298:dbl)
                      n125 = Divide(x=w293, y=w295) -> (x/y=w297:dbl)
                      n126 = Send Notification(notification=TRUE, notifier=w312, error in (no error)=w309) -> (notifier out=w310:refnum<notifier>, error out=w308:errorcluster)
                      n127 = Multiply(x=w298, y=w296) -> (x*y=w292:dbl)
                      n128 = Multiply(x=w297, y=w296) -> (x*y=w291:dbl)
                      n129 = Insert Into Array(array=w306, new element=w292) -> (w290:dbl[])  [unwired: 1 in]
                      n130 = local write "LD array disc"(w290) -> ()
                      n131 = Insert Into Array(array=w305, new element=w291) -> (w302:dbl[])  [unwired: 1 in]
                      n132 = local write "LD error array disc"(w302) -> ()
                      n133 = local read "dPhase array"() -> (w323:dbl[])
                      n134 = local read "LD error array"() -> (w317:dbl[])
                      n135 = local read "Phase array"() -> (w322:dbl[])
                      n136 = local read "2f Frequency (Hz)"() -> (w329:dbl)
                      n137 = local read "Frequency array"() -> (w328:dbl[])
                      n138 = local read "LD array"() -> (w319:dbl[])
                      n139 = Insert Into Array(array=w328, new element=w329) -> (w304:dbl[])  [unwired: 1 in]
                      n140 = Bundle("Frequency array"=w304, "LD array disc"=w290) -> (w303:T11)  [unwired: 1 in]
                      n141 = call "XY error bars_diag.vi"("XY plot"=w303, "Yerror"=w302) -> ("Y error bars"=w300:cluster{dbl[], dbl[]})  [unwired: 6 in, 2 out]
                      n142 = Insert Into Array(array=w317, new element=w315) -> (w318:dbl[])  [unwired: 1 in]
                      n143 = Insert Into Array(array=w322, new element=w314) -> (w324:dbl[])  [unwired: 1 in]
                      n144 = Insert Into Array(array=w323, new element=w313) -> (w326:dbl[])  [unwired: 1 in]
                      n145 = Insert Into Array(array=w319, new element=w316) -> (w320:dbl[])  [unwired: 1 in]
                      n146 = local write "LD error array"(w318) -> ()
                      n147 = local write "LD array"(w320) -> ()
                      n148 = local write "Frequency array"(w304) -> ()
                      n149 = Bundle("Frequency array"=w304, "LD array"=w320) -> (w321:T12)  [unwired: 1 in]
                      n150 = local write "Phase array"(w324) -> ()
                      n151 = local write "dPhase array"(w326) -> ()
                      n152 = call "XY error bars_diag.vi"("XY plot"=w321, "Yerror"=w318) -> ("Y error bars"=w301:cluster{dbl[], dbl[]})  [unwired: 6 in, 2 out]
                      n153 = Bundle("Frequency array"=w304, "Phase array"=w324) -> (w325:T13)  [unwired: 1 in]
                      n154 = call "XY error bars_diag.vi"("XY plot"=w325, "Yerror"=w326) -> ("Y error bars"=→"MLD Phase":cluster{dbl[], dbl[]})  [unwired: 6 in, 2 out]
                      n155 = Build Array(w301, w300) -> (→"MLD Amplitude (mV/V)":cluster{dbl[], dbl[]}[])
                      "LD(cont/disc)" <- w307
                    }
                  }
                  n156 = while {
                    tunnel: w215 -> [w245]
                    tunnel: [w237] -> w218
                    tunnel: w211 -> [w244]
                    tunnel: w210 -> [w243]
                    tunnel: [w242] -> w209
                    stop <- w238 stop-if-true
                    n157 = Get Notifier Status(notifier=w244, error in (no error)=w243) -> (current notification=w239:bool, error out=w242:errorcluster)  [unwired: 3 out]
                    n158 = local read "DC Voltage (V) 2"() -> (w241:dbl)
                    n159 = local read "level B"() -> (w233:dbl)
                    n160 = local read "level A"() -> (w234:dbl)
                    n161 = local read "AC?"() -> (w224:bool)
                    n162 = local read "Reference Signal"() -> (w247:tag)
                    n163 = local read "V/div A"() -> (w236:dbl)
                    n164 = local read "LD Signal"() -> (w246:tag)
                    n165 = local read "V/div B"() -> (w235:dbl)
                    n166 = call "fast_scope_diag.vi"("Sensitivity"=T5."-10V..10V", "Reference Signal"=w247, "AC?"=w224, "mean"=w241, "LD Signal"=w246, "V/div"=w236, "error in (no error)"=w245, "Max frequency (Hz)"=200.0, "V/div in B"=w235, "level B"=w233, "Refresh in (s)"=1.0, "level A"=w234) -> ("levelA"=w230:dbl, "levelB"=w229:dbl, "Unbalanced"=w228:bool, "1f Peak (mv/V)"=w222:dbl, "MLD SA (mV/V)"=w221:dbl, "Scale Max"=w225:dbl, "Scale Min"=w227:dbl, "Frequency"=w223:dbl, "Spectrum"=w231:cluster{"f0":dbl, "df":dbl, "magnitude":dbl[]}, "V/div out"=w226:dbl, "Array"=w232:waveform(dbl)[], "error out"=w237:errorcluster)  [unwired: 4 in]
                    n167 = local write "1f SA (mV/V)"(w222) -> ()
                    n168 = local write "Spectrum (mVRMS/Vdc)"(w231) -> ()
                    n169 = local write "Oscilloscope"(w232) -> ()
                    n170 = local write "levelB"(w229) -> ()
                    n171 = local write "levelA"(w230) -> ()
                    n172 = local write "2f Frequency (Hz)"(w223) -> ()
                    n173 = property on="Oscilloscope" class="WFChart (strict)"("YScale.Increment"=w226, "YScale.Maximum"=w225, "YScale.Minimum"=w227) -> ()  [unwired: 2 in, 2 out]
                    n174 = local write "error out"(w237) -> ()
                    n175 = Not(x=w228) -> (.not. x?=w240:bool)
                    n176 = local write "Signal Balance"(w228) -> ()
                    n177 = And(x=w240, y=w239) -> (x .and. y?=w238:bool)
                    n178 = local write "MLD SA (mV/V)"(w221) -> ()
                  }
                  n179 = Merge Errors(w212, w209) -> (w213:errorcluster)
                  n180 = Release Notifier(notifier=w214, error in (no error)=w213) -> ()  [unwired: 1 in, 3 out]
                  n181 = Merge Errors(w219, w218) -> (w217:errorcluster)
                }
                frame "Save" {
                  n182 = local read "dLock_in (mV/V)"() -> (w336:dbl)
                  n183 = local read "Lock_in (mV/V)"() -> (w337:dbl)
                  n184 = local read "SA 2f (mv/V)"() -> (w338:dbl)
                  n185 = local read "SA 1f (mv/V)"() -> (w339:dbl)
                  n186 = local read "Unbalanced?"() -> (w331:bool)
                  n187 = local read "Phase  dev (deg)"() -> (w349:dbl)
                  n188 = local read "Dc standard deviation"() -> (w347:dbl)
                  n189 = local read "2f Frequency (Hz)"() -> (w342:dbl)
                  n190 = local read "dMLD (mV/V)"() -> (w340:dbl)
                  n191 = local read "MLD (mV/V)"() -> (w341:dbl)
                  n192 = local read "Phase (deg)"() -> (w350:dbl)
                  n193 = local read "Dc mean"() -> (w348:dbl)
                  n194 = Boolean To (0,1)(Boolean=w331) -> (0, 1=w333:i16)
                  n195 = To Double Precision Float(number=w333) -> (double precision float=w332:dbl)
                  n196 = Build Array(w342, w341, w340, w339, w338, w337, w336, w350, w349, w348, w347, w332) -> (w345:dbl[])
                  n197 = global read "Global 1_diag.vi" "Measurement File"() -> (w346:path)
                  n198 = call-poly <vilib>:"Write To Spreadsheet File.vi"("format (%.3f)"="%g", "append to file? (new file:F)"=TRUE, "1D data"=w345, "file path (dialog if empty)"=w346) -> ()  [unwired: 4 in, 1 out]
                  n199 = local read "Last Step?"() -> (w330:bool)
                  n200 = case shown="True" w330 {
                    tunnel: [State_machine_enum."Measure" State_machine_enum."Finished"] -> w334
                    frame False {
                    }
                    frame True {
                    }
                  }
                }
                frame "Finished" {
                  n201 = local read "Last Step?"() -> (w354:bool)
                }
              }
              n202 = local read "Stopped"() -> (w101:bool)
              n203 = Compound Arithmetic op=OR(w103, w102, w101) -> (w100:bool)
              "Actual State" <- w104
            }
          }
          frame #2 {
            # "Terminating"
            n204 = local read "Stopped"() -> (w357:bool)
            n205 = case shown="False" w357 {
              tunnel: w358 -> [w366 _]
              tunnel: [w365 w370] -> w355
              tunnel: w356 -> [w364 w370]
              frame False {
                n206 = local write "Reset?"(TRUE ("Reset?")) -> ()
                n207 = local write "Actual Task"("Measurement finished" ("Actual Task")) -> ()
                n208 = local read "Motor Voltage (V)"() -> (w359:dbl)
                n209 = local read "Motor Channel"() -> (w362:tag)
                n210 = call "gradual_motorset_diag.vi"("Initial Voltage (V)"=w359, "error in (no error)"=w364, "Steps"=500.0, "Next Voltage (V)"=0.0 ("Numeric"), "Physical Channel"=w362) -> ("error out"=w363:errorcluster)  [unwired: 6 in]
                n211 = Merge Errors(w366, w363) -> (w365:errorcluster)
              }
              frame True {
                n212 = local write "Stopped"(FALSE ("Stopped")) -> ()
              }
            }
            n213 = local write "error out"(w355) -> ()
          }
        }
      }
      frame "stop" {
        n214 = call <vilib>:"Three Button Dialog.vi"("Window Title (\"\")"="Stop Measurement" ("Window Title (\"\")"), "Right Button Text (\"Cancel\")"="Continue" ("Right Button Text (\"Cancel\")"), "Center Button Text (\"No\")"="Pause" ("Right Button Text (\"Cancel\")"), "Left Button Text (\"Yes\")"="Stop and Reset" ("Left Button Text (\"Yes\")"), "message"="Would You like to stop measurement?") -> ("Which Button?"=w374:T9)  [unwired: 6 in]
        n215 = case shown="\"Center Button\"" w374 {
          tunnel: w373 -> [w382 w402 w434]
          tunnel: [w381 w401 w434] -> w372
          tunnel: w371 -> [_ w400 w433]
          frame "Left Button", Default {
            # "Stop and reset"
            n216 = local write "Reset?"(TRUE ("Reset?")) -> ()
            n217 = local read "Motor Channel"() -> (w383:tag)
            n218 = global read "Global 1_diag.vi" "Measurement File"() -> (w385:path)
            n219 = call "motor_control_voltage.vi"("Error In"=w382, "Numeric"=0.0, "Physical Channel"=w383) -> ("error out"=w381:errorcluster)  [unwired: 8 in]
            n220 = Not A Number/Path/Refnum?(number/path/refnum=w385) -> (NaN/Path/Refnum?=w386:bool)
            n221 = Empty String/Path?(string/path=w385) -> (empty?=w387:bool)
            n222 = Or(x=w386, y=w387) -> (x .or. y?=w388:bool)
            n223 = case shown="False" w388 {
              tunnel: w385 -> [w389 _]
              frame False {
                n224 = local read "Phase  dev (deg)"() -> (w392:dbl)
                n225 = local read "Dc standard deviation"() -> (w390:dbl)
                n226 = local read "2f Frequency (Hz)"() -> (w396:dbl)
                n227 = local read "dMLD (mV/V)"() -> (w394:dbl)
                n228 = local read "MLD (mV/V)"() -> (w395:dbl)
                n229 = local read "Phase (deg)"() -> (w393:dbl)
                n230 = local read "Dc mean"() -> (w391:dbl)
                n231 = Build Array(w396, w395, w394, w393, w392, w391, w390) -> (w399:dbl[])
                n232 = call-poly <vilib>:"Write To Spreadsheet File.vi"("format (%.3f)"="%g", "append to file? (new file:F)"=TRUE, "1D data"=w399, "file path (dialog if empty)"=w389) -> ()  [unwired: 4 in, 1 out]
              }
              frame True {
              }
            }
          }
          frame "Center Button" {
            # "Pause"
            n233 = local write "Reset?"(FALSE ("Reset?")) -> ()
            n234 = local write "Stopped"(FALSE ("Stopped")) -> ()
            n235 = local write "Actual Task"("Paused" ("Actual Task")) -> ()
            n236 = while {
              tunnel: w402 -> [w424]
              tunnel: [w423] -> w401
              tunnel: w400 -> [w420]
              stop <- w421 stop-if-true
              n237 = local read "Reference Signal"() -> (w428:tag)
              n238 = local read "LD Signal"() -> (w429:tag)
              n239 = Get Queue Status(queue=w420) -> (# elements in queue=w422:i32)  [unwired: 2 in, 7 out]
              n240 = local read "DC Voltage (V) 2"() -> (w419:dbl)
              n241 = local read "AC?"() -> (w418:bool)
              n242 = Greater Than 0?(x=w422) -> (x > 0?=w421:bool)
              n243 = local read "V/div B"() -> (w416:dbl)
              n244 = local read "level A"() -> (w415:dbl)
              n245 = local read "level B"() -> (w414:dbl)
              n246 = local read "V/div A"() -> (w417:dbl)
              n247 = call "fast_scope_diag.vi"("Sensitivity"=T5."-10V..10V", "Reference Signal"=w428, "AC?"=w418, "mean"=w419, "LD Signal"=w429, "V/div"=w417, "error in (no error)"=w424, "Max frequency (Hz)"=200.0, "V/div in B"=w416, "level B"=w414, "Refresh in (s)"=1.0, "level A"=w415) -> ("levelA"=w413:dbl, "levelB"=w412:dbl, "Unbalanced"=w406:bool, "Scale Max"=w409:dbl, "Scale Min"=w408:dbl, "Spectrum"=w410:cluster{"f0":dbl, "df":dbl, "magnitude":dbl[]}, "V/div out"=w407:dbl, "Array"=w411:waveform(dbl)[], "error out"=w423:errorcluster)  [unwired: 4 in, 3 out]
              n248 = local write "levelA"(w413) -> ()
              n249 = local write "levelB"(w412) -> ()
              n250 = local write "Spectrum (mVRMS/Vdc)"(w410) -> ()
              n251 = local write "Signal Balance"(w406) -> ()
              n252 = local write "Oscilloscope"(w411) -> ()
              n253 = property on="Oscilloscope" class="WFChart (strict)"("YScale.Increment"=w407, "YScale.Maximum"=w409, "YScale.Minimum"=w408) -> ()  [unwired: 2 in, 2 out]
            }
          }
          frame "Right Button" {
            # "Continue"
            n254 = Enqueue Element(queue=w433, element=User_buttons_enum."start") -> ()  [unwired: 2 in, 3 out]
            n255 = local write "Stopped"(FALSE ("Stopped")) -> ()
            "Reset?" <- FALSE ("Reset?")
          }
        }
      }
      frame "exit" {
        # "This will stop the consumer loop, thus exit this\nportion of the program."
      }
      frame "New" {
        n256 = call "Create_file_diag.vi"("error in (no error)"=w439) -> ("error out"=w438:errorcluster, "Measurement File out"=w437:path)  [unwired: 9 in]
        n257 = local write "Measurement File"(w437) -> ()
      }
      frame "Scope" {
        w463 = 10123 items=["Finite Samples"=10178, "Continuous Samples"=10123, "Hardware Timed Single Point"=12522]  # sample mode
        w470 = FALSE  # auto cleanup
        n258 = Divide(x=1.0, y="rate") -> (x/y=→"dt":dbl)
        n259 = local read "DC Voltage DAQ"() -> (w440:tag)
        n260 = call <vilib>:"DAQmx Create Task.vi"("auto cleanup"=w470, "error in"=w447) -> ("task out"=w446:refnum<k21>, "error out"=w445:errorcluster)  [unwired: 12 in]
        n261 = local read "Reference Signal"() -> (w472:tag)
        n262 = call-poly <vilib>:"DAQmx Create Virtual Channel.vi"("task in"=w446, "maximum value"=10.0, "minimum value"=-10.0, "physical channels"=w440, "error in"=w445) -> ("task out"=w444:refnum<k21>, "error out"=w443:errorcluster)  [unwired: 9 in]
        n263 = call-poly <vilib>:"DAQmx Create Virtual Channel.vi"("task in"=w444, "maximum value"=10.0, "minimum value"=-10.0, "physical channels"=w472, "error in"=w443) -> ("task out"=w466:refnum<k21>, "error out"=w467:errorcluster)  [unwired: 9 in]
        n264 = local read "LD Signal"() -> (w471:tag)
        n265 = case shown="\"-1V..1V\", Default" "Sensitivity" {
          tunnel: [-1.0 ("maximum value") -1.25 ("maximum value") -2.0 ("maximum value") -2.5 ("maximum value") -4.0 ("maximum value") -5.0 ("maximum value") -10.0 ("maximum value")] -> w461
          tunnel: [1.0 ("maximum value") 1.25 ("maximum value") 2.0 ("maximum value") 2.5 ("maximum value") 4.0 ("maximum value") 5.0 ("maximum value") 10.0 ("maximum value")] -> w460
          frame "-1V..1V", Default {
          }
          frame "-1.25V..1.25V" {
          }
          frame "-2V..2V" {
          }
          frame "-2.5V..2.5V" {
          }
          frame "-4V..4V" {
          }
          frame "-5V..5V" {
          }
          frame "-10V..10V" {
          }
        }
        n266 = call-poly <vilib>:"DAQmx Create Virtual Channel.vi"("task in"=w466, "maximum value"=w460, "minimum value"=w461, "physical channels"=w471, "error in"=w467) -> ("task out"=w464:refnum<k21>, "error out"=w465:errorcluster)  [unwired: 9 in]
        n267 = call-poly <vilib>:"DAQmx Timing.vi"("task/channels in"=w464, "sample mode"=w463, "samples per channel"="samples per channel", "rate"="rate", "error in"=w465) -> ("task out"=w451:refnum<k21>, "error out"=w449:errorcluster)  [unwired: 9 in]
        n268 = property class="DAQmx Channel"(reference=w451, error in=w449, "AI.UsbXferReqCount"=u32 1) -> (reference out=w450:refnum<k21>, error out=w448:errorcluster)
        n269 = while {
          tunnel: [w505] -> w454
          tunnel: w448 -> [w490]
          tunnel: w450 -> [w495]
          tunnel: "samples per channel" -> [w494]
          tunnel: [w492] -> w455
          stop <- w507 stop-if-true
          n270 = Obtain Queue(element data type=dbl[][] [] ("data")) -> (queue out=w511:refnum<queue>)  [unwired: 4 in, 2 out]
          n271 = while {
            tunnel: w511 -> [w519]
            shift-right: [w513] -> w489
            shift-left: dbl[][] [] ("element data type") -> [w520]
            i -> [w516]
            stop <- w512 stop-if-true
            n272 = Equal?(x=0, y=w516) -> (x = y?=w514:bool)
            n273 = Dequeue Element(queue=w519) -> (element=w518:dbl[][], error out=w517:errorcluster)  [unwired: 2 in, 2 out]
            n274 = case shown="No Error" w517 {
              tunnel: w518 -> [w523 _]
              tunnel: w520 -> [w555 w586]
              tunnel: w514 -> [w554 _]
              tunnel: [w533 w586] -> w513
              tunnel: [FALSE TRUE] -> w512
              frame No Error {
                n275 = Transpose 2D Array(2D array=w523) -> (transposed array=w522:dbl[][])
                n276 = Index Array(array=w522, index (col)=2) -> (element=w521:dbl[])  [unwired: 1 in]
                n277 = Index Array(array=w522, index (col)=1) -> (element=w527:dbl[])  [unwired: 1 in]
                n278 = Build Array(w527, w521) -> (w525:dbl[][])
                n279 = Transpose 2D Array(2D array=w525) -> (transposed array=w524:dbl[][])
                n280 = Insert Into Array(array=w555, new element=w524) -> (w526:dbl[][])  [unwired: 2 in]
                n281 = local read "dt"() -> (w540:dbl)
                n282 = call "Scopeset_diag.vi"("Ref_MLD measurement"=w524, "V/div in B"="V/div B", "AC?"="AC?", "V/div in A"="V/div A", "level B"="level B", "level A"="level A", "dt"=w540) -> ("UP"=→"Up":bool, "Down"=→"Down":bool, "V/div out"=w563:dbl, "Ref_MLD_triggered"=w556:dbl[][], "levelB"=→"levelB":dbl, "Scale Max"=w565:dbl, "Scale Min"=w564:dbl, "levelA"=→"levelA":dbl, "Array"=→"Oscilloscope":waveform(dbl)[], "Frequency"=w537:dbl)  [unwired: 1 in, 2 out]
                n283 = property on="Oscilloscope" class="WFChart (strict)"("YScale.Increment"=w563, "YScale.Maximum"=w565, "YScale.Minimum"=w564) -> ()  [unwired: 2 in, 2 out]
                n284 = local write "2f Frequency (Hz)"(w537) -> ()
                n285 = local write "2f Frequency (Hz)"(w537) -> ()
                n286 = case shown="True" w554 {
                  tunnel: w556 -> [_ w584]
                  tunnel: w526 -> [w583 _]
                  tunnel: [w583 w584] -> w533
                  frame False {
                  }
                  frame True {
                  }
                }
                n287 = Index Array(array=w533, index (col)=0 ("disabled index (col)")) -> (element=w547:dbl[])  [unwired: 1 in]
                n288 = Index Array(array=w522, index (col)=0) -> (element=w532:dbl[])  [unwired: 1 in]
                n289 = Index Array(array=w533, index (col)=1 ("disabled index (col)")) -> (element=w548:dbl[])  [unwired: 1 in]
                n290 = Bundle By Name("Y"=w547, "dt"=w540) -> (w550:waveform(dbl))  [unwired: 1 in]
                n291 = Bundle By Name("Y"=w548, "dt"=w540) -> (w551:waveform(dbl))  [unwired: 1 in]
                n292 = call-poly <vilib>:"Mean.vi"("X"=w532) -> ("mean"=w531:dbl)  [unwired: 1 out]
                "DC Voltage (V)" <- w531
                n293 = Build Array(w551, w550) -> (→"Waveform Graph":waveform(dbl)[])
                n294 = local write "DC Voltage (V) 2"(w531) -> ()
                n295 = case shown="False" "Lock In" {
                  tunnel: w531 -> [_ w568]
                  frame False {
                  }
                  frame True {
                    n296 = local read "Lock-in-Amplifier VISA"() -> (w572:refnum<visa-resource-name>)
                    n297 = call "Lock_in_single_meas.vi"("Lock-in-Amplifier VISA"=w572) -> ("Lockin_ampl"=w570:dbl, "Freq"=→"Lockin_freq":dbl)  [unwired: 7 in, 2 out]
                    n298 = xnode "LIA calc"("X1"=w570, "X2"=w568) -> ("Result"=→"MLD LIA (mV/V)":dbl)  [unwired: 1 in, 1 out]
                  }
                }
                n299 = Index Array(array=w533, index (col)=1 ("disabled index (col)")) -> (element=w546:dbl[])  [unwired: 1 in]
                n300 = Bundle By Name("Y"=w546, "dt"=w540) -> (w530:waveform(dbl))  [unwired: 1 in]
                n301 = call "Fast_spectrum_analyzer_diag.vi"("mean"=w531, "Waveform"=w530, "Frequency"=w537) -> ("error out"=w545:errorcluster, "MLD SA (mV/V)"=w539:dbl, "Spectrum (mV/V)"=→"Spectrum (mVRMS/Vdc)":cluster{"f0":dbl, "df":dbl, "magnitude":dbl[]}, "1f Peak (mv/V)"=w538:dbl)  [unwired: 5 in]
                n302 = local write "MLD SA (mV/V)"(w539) -> ()
                n303 = local write "1f SA (mV/V)"(w538) -> ()
                n304 = local write "error out"(w545) -> ()
              }
              frame Error {
              }
            }
          }
          n305 = while {
            tunnel: [w602] -> w492
            shift-right: [w587] -> w493
            shift-left: w490 -> [w603]
            tunnel: [w599] -> _
            tunnel: w511 -> [w598]
            tunnel: [w596] -> w510
            tunnel: w495 -> [w595]
            tunnel: w494 -> [w594]
            tunnel: ["stop"] -> w506
            i -> [w593]
            stop <- w599 stop-if-true
            w600 = 10.0  # timeout (s)
            n306 = Subtract(x="Refresh in (s)", y=i8 2) -> (x-y=w591:i8)
            n307 = Less?(x=w591, y=w593) -> (x < y?=w592:bool)
            n308 = call-poly <vilib>:"DAQmx Read.vi"("task/channels in"=w595, "number of samples per channel"=w594, "timeout"=w600, "error in"=w603) -> ("task out"=w602:refnum<k21>, "data"=w597:dbl[][], "error out"=w587:errorcluster)  [unwired: 9 in]
            n309 = Unbundle By Name(w587) -> ("status"=w601:bool)
            n310 = local write "error out"(w587) -> ()
            n311 = Enqueue Element(queue=w598, element=w597) -> (queue out=w596:refnum<queue>)  [unwired: 2 in, 2 out]
            n312 = Compound Arithmetic op=OR(w601, "stop", w592) -> (w599:bool)
            "result" <- w599
          }
          n313 = Merge Errors(w493) -> (w504:errorcluster)
          n314 = Release Queue(queue=w510, error in (no error)=w504) -> (error out=w505:errorcluster)  [unwired: 1 in, 2 out]
          n315 = local read "DC Voltage (V) 2"() -> (w487:dbl)
          n316 = local read "Refresh in (s)"() -> (w500:i8)
          n317 = Array Size(array=w489) -> (size(s)=w498:i32[])
          n318 = Transpose 2D Array(2D array=w489) -> (transposed array=w488:dbl[][])
          n319 = Index Array(array=w498, index=0) -> (element=w499:i32)
          n320 = local read "rate"() -> (w502:dbl)
          n321 = local read "dt"() -> (w503:dbl)
          n322 = local read "Second Harmonic"() -> (w497:bool)
          n323 = call "Lockin_Amplifier_diag_fast.vi"("Sampling frequency"=w502, "Number of samples"=w499, "dt"=w503, "Second"=w497, "Ref_MLD measurement"=w488, "mean"=w487, "Refresh in (s)"=w500) -> ("Result"=→"dLD_RMS":dbl, "Result 2"=w491:dbl)  [unwired: 3 in]
          n324 = local write "MLD Sim. LIA (mV/V)"(w491) -> ()
          n325 = Compound Arithmetic op=OR(w506, w505) -> (w507:bool)
        }
        n326 = call <vilib>:"DAQmx Clear Task.vi"("task in"=w455, "error in"=w454) -> ("error out"=w453:errorcluster)  [unwired: 13 in]
      }
    }
    n327 = Unbundle By Name(w15) -> ("status"=w14:bool)
    n328 = Or(x=w14, y=w13) -> (x .or. y?=w12:bool)
  }
  n329 = while {
    shift-right: [w606] -> w7
    shift-left: w10 -> [w609]
    tunnel: w3 -> [w610]
    tunnel: [w604] -> w8
    stop <- w607 stop-if-true
    # "This loop is the producer loop."
    n330 = event shown="[10] \"Convert parasiteno\": Value Change" {
      selector: _ -> [_ _ _ _ _ _ _ _ _ _ _]
      dyn-events: _ -> [_ _ _ _ _ _ _ _ _ _ _]
      timeout: _ -> [_ _ w622 _ _ _ _ _ _ _ _]
      tunnel: w610 -> [w615 w620 w624 w633 w638 _ _ _ _ _ _]
      tunnel: w609 -> [w614 w621 w627 w632 w637 w642 _ _ _ _ _]
      tunnel: [w613 w618 w626 w630 w635 w641 _ _ _ _ _] -> w606
      tunnel: [_ _ "EXIT" _ _ _ _ _ _ _ _] -> w608
      tunnel: [w612 w619 w625 w631 w636 _ _ _ _ _ _] -> w604
      tunnel: [_ _ w622 _ _ _ _ _ _ _ _] -> _
      event "Start Measurement Button": Value Change {
        n331 = event-data() -> ()  [unwired: 1 in, 1 out]
        n332 = Enqueue Element(queue=w615, element=User_buttons_enum."start", error in (no error)=w614) -> (queue out=w612:refnum<queue>, error out=w613:errorcluster)  [unwired: 1 in, 1 out]
      }
      event "Stop Measurement": Value Change {
        n333 = event-data() -> ()  [unwired: 1 in, 1 out]
        n334 = Enqueue Element(queue=w620, element=User_buttons_enum."stop", error in (no error)=w621) -> (queue out=w619:refnum<queue>, error out=w618:errorcluster)  [unwired: 1 in, 1 out]
        "Stopped" <- TRUE
      }
      event "EXIT": Value Change {
        n335 = event-data() -> ()  [unwired: 1 in, 1 out]
        n336 = Enqueue Element(queue=w624, element=User_buttons_enum."exit", error in (no error)=w627) -> (queue out=w625:refnum<queue>, error out=w626:errorcluster)  [unwired: 1 in, 1 out]
      }
      event "New File": Value Change {
        n337 = event-data() -> ()  [unwired: 1 in, 1 out]
        n338 = Enqueue Element(queue=w633, element=User_buttons_enum."New", error in (no error)=w632) -> (queue out=w631:refnum<queue>, error out=w630:errorcluster)  [unwired: 1 in, 1 out]
      }
      event "Start Scope": Value Change {
        n339 = event-data() -> ()  [unwired: 1 in, 1 out]
        n340 = Enqueue Element(queue=w638, element=User_buttons_enum."Scope", error in (no error)=w637) -> (queue out=w636:refnum<queue>, error out=w635:errorcluster)  [unwired: 1 in, 1 out]
      }
      event "Constant Motor Voltage": Value Change {
        n341 = event-data() -> ("OldVal"=w640:dbl)  [unwired: 1 in]
        n342 = local write "Motor Voltage (V)"("Constant Motor Voltage") -> ()
        n343 = local read "Motor Channel"() -> (w644:tag)
        n344 = call "gradual_motorset_diag.vi"("Initial Voltage (V)"=w640, "error in (no error)"=w642, "Steps"=500.0, "Next Voltage (V)"="Constant Motor Voltage", "Physical Channel"=w644) -> ("error out"=w641:errorcluster)  [unwired: 6 in]
      }
      event "Convert dT": Value Change {
        n345 = event-data() -> ()  [unwired: 1 in, 1 out]
        n346 = local read "dT/T (%)"() -> (w653:dbl)
        n347 = local read "Dilution"() -> (w647:dbl)
        n348 = Multiply(x=w653, y=1200.0) -> (x*y=w654:dbl)
        n349 = Divide(x=w653, y=0.0012) -> (x/y=w646:dbl)
        n350 = Multiply(x=w647, y=w646) -> (x*y=w645:dbl)
        n351 = local write "Undiluted cc.\n (ng/ml)"(w645) -> ()
        n352 = local write "MLD (mV/V)"(w654) -> ()
        n353 = Multiply(x=w645, y=2.0) -> (x*y=w650:dbl)
        n354 = Multiply(x=w650, y=2e-05) -> (x*y=w648:dbl)
        n355 = local write "Undiluted \nParasitemia (%)"(w648) -> ()
        n356 = local write "Parasites/ul\nof Blood"(w650) -> ()
      }
      event "Convert mld": Value Change {
        n357 = event-data() -> ()  [unwired: 1 in, 1 out]
        n358 = local read "MLD (mV/V)"() -> (w658:dbl)
        n359 = local read "Dilution"() -> (w660:dbl)
        n360 = Divide(x=w658, y=1200.0) -> (x/y=w657:dbl)
        n361 = Divide(x=w657, y=0.0012) -> (x/y=w659:dbl)
        n362 = Multiply(x=w660, y=w659) -> (x*y=w656:dbl)
        n363 = local write "Undiluted cc.\n (ng/ml)"(w656) -> ()
        n364 = local write "dT/T (%)"(w657) -> ()
        n365 = Multiply(x=w656, y=2.0) -> (x*y=w663:dbl)
        n366 = Multiply(x=w663, y=2e-05) -> (x*y=w661:dbl)
        n367 = local write "Undiluted \nParasitemia (%)"(w661) -> ()
        n368 = local write "Parasites/ul\nof Blood"(w663) -> ()
      }
      event "Convert cc": Value Change {
        n369 = event-data() -> ()  [unwired: 1 in, 1 out]
        n370 = local read "Undiluted cc.\n (ng/ml)"() -> (w667:dbl)
        n371 = local read "Dilution"() -> (w673:dbl)
        n372 = Divide(x=w667, y=w673) -> (x/y=w672:dbl)
        n373 = Multiply(x=w667, y=2.0) -> (x*y=w674:dbl)
        n374 = Multiply(x=0.0012 ("y"), y=w672) -> (x*y=w670:dbl)
        n375 = local write "Parasites/ul\nof Blood"(w674) -> ()
        n376 = local write "dT/T (%)"(w670) -> ()
        n377 = Multiply(x=w674, y=2e-05) -> (x*y=w677:dbl)
        n378 = local write "Undiluted \nParasitemia (%)"(w677) -> ()
        n379 = Multiply(x=1200.0 ("y"), y=w670) -> (x*y=w668:dbl)
        n380 = local write "MLD (mV/V)"(w668) -> ()
      }
      event "Convert parasitemia": Value Change {
        n381 = event-data() -> ()  [unwired: 1 in, 1 out]
        n382 = local read "Undiluted \nParasitemia (%)"() -> (w684:dbl)
        n383 = Divide(x=w684, y=2e-05) -> (x/y=w687:dbl)
        n384 = local read "Dilution"() -> (w688:dbl)
        n385 = Divide(x=w687, y=2.0) -> (x/y=w679:dbl)
        n386 = Divide(x=w679, y=w688) -> (x/y=w678:dbl)
        n387 = Multiply(x=0.0012 ("y"), y=w678) -> (x*y=w682:dbl)
        n388 = local write "dT/T (%)"(w682) -> ()
        n389 = local write "Undiluted cc.\n (ng/ml)"(w679) -> ()
        n390 = local write "Parasites/ul\nof Blood"(w687) -> ()
        n391 = Multiply(x=1200.0 ("y"), y=w682) -> (x*y=w680:dbl)
        n392 = local write "MLD (mV/V)"(w680) -> ()
      }
      event "Convert parasiteno": Value Change {
        n393 = event-data() -> ()  [unwired: 1 in, 1 out]
        n394 = local read "Parasites/ul\nof Blood"() -> (w691:dbl)
        n395 = Multiply(x=w691, y=2e-05) -> (x*y=w699:dbl)
        n396 = local read "Dilution"() -> (w698:dbl)
        n397 = Divide(x=w691, y=2.0) -> (x/y=w690:dbl)
        n398 = local write "Undiluted \nParasitemia (%)"(w699) -> ()
        n399 = Divide(x=w690, y=w698) -> (x/y=w689:dbl)
        n400 = Multiply(x=0.0012 ("y"), y=w689) -> (x*y=w694:dbl)
        n401 = local write "dT/T (%)"(w694) -> ()
        n402 = local write "Undiluted cc.\n (ng/ml)"(w690) -> ()
        n403 = Multiply(x=1200.0 ("y"), y=w694) -> (x*y=w692:dbl)
        n404 = local write "MLD (mV/V)"(w692) -> ()
      }
    }
    n405 = Unbundle By Name(w606) -> ("status"=w605:bool)
    n406 = Or(x=w605, y=w608) -> (x .or. y?=w607:bool)
  }
  n407 = local read "Sensitivity"() -> (w1:T5)
  n408 = case shown="\"-1V..1V\", Default" w1 {
    tunnel: [-1.0 ("maximum value") -1.25 ("maximum value") -2.0 ("maximum value") -2.5 ("maximum value") -4.0 ("maximum value") -5.0 ("maximum value") -10.0 ("maximum value")] -> _
    tunnel: [1.0 ("maximum value") 1.25 ("maximum value") 2.0 ("maximum value") 2.5 ("maximum value") 4.0 ("maximum value") 5.0 ("maximum value") 10.0 ("maximum value")] -> _
    frame "-1V..1V", Default {
    }
    frame "-1.25V..1.25V" {
    }
    frame "-2V..2V" {
    }
    frame "-2.5V..2.5V" {
    }
    frame "-4V..4V" {
    }
    frame "-5V..5V" {
    }
    frame "-10V..10V" {
    }
  }
  n409 = Merge Errors(w7, w6) -> (w5:errorcluster)
  n410 = Release Queue(queue=w8, error in (no error)=w5) -> ()  [unwired: 1 in, 3 out]
